vi "Text control 2 v1.9.vi"() -> ()   [LabVIEW 2016]
panel:
  out "Total iterations":i32
  out "Line running":i32
  in  "byte count":u32=64
  in  "Serial Settings:Serial End Mode for Reads":u16(ring)=2 items=["None", "LastBit", "TermChar"]
  in  "Timeout (ms)":u32=10000
  in  "Enable Termination\nChar (T)":bool=TRUE
  in  "Termination char\n(0xA = '\\n' = LF)\n(0xD = '\\r' = CR)":u8=13 format="%.0x"
  in  "flow control":u16(ring) items=["None"=0, "XON/XOFF"=1, "RTS/CTS"=2, "DTR/DSR"=4]
  in  "stop bits":u16(ring)=10 items=["1.0"=10, "1.5"=15, "2.0"=20]
  in  "parity":u16(ring) items=["None", "Odd", "Even", "Mark", "Space"]
  in  "data bits":u16=8 min=5 max=8 step=1
  in  "VISA resource name":refnum<visa-resource-name>="COM6"
  in  "baud rate":u32=9600
  out "Serial output":string
  out "error out":errorcluster
  in  "Units":bool
  out "Elapsed Time":dbl caption="Elapsed Time (s)"
  out "Ion vs time":cluster{"Y data in":dbl[], "X data in":dbl[]}[](graph)
  out "Ig":dbl format="%.2e"
  out "Id":dbl format="%.2e"
  out "Is":dbl format="%.2e"
  out "I vs Vg":cluster{"Y data in":dbl[], "X data in":dbl[]}[](graph)
  in  "Panel Controls 2":T1={"Emergency Stop"=refnum, "TransGraph Max"=1e-05, "Text/Graph (text=false)"=TRUE, "TransGraph Min"=1e-11} {"TransGraph Min" format="%.2e"; "TransGraph Max" format="%.2e"}
  out "Command running:":string="#output s 0 0 0 -0.008 0.008 0.002"
  in  "Standby":T2
  in  "Full Reset":bool
  in  "SMU4":cluster{"on/off":bool, "Voltage":dbl} {"Voltage" min=-100.0 max=100.0 format="%.2f"}
  in  "Source/Drain Range":u8(slide)=6 max=11 scale=0.0..11.0
  in  "Source/Drain\nRange mode":u16(ring) items=["Auto", "Limited", "Fixed"]
  in  "Gate Range":u8(slide)=6 max=11 scale=0.0..11.0
  in  "Gate Range\nmode":u16(ring) items=["Auto", "Limited", "Fixed"]
  in  "Gate":T3={"Gate Start"=0.0, "Gate Stop"=2.0, "Gate Step (linear only)"=1.0, "Gate Compliance"=0.0001, "Gate PComp"=0.0, "Range mode"=0, "Range"=6} {"Range" max=11 scale=0.0..11.0; "Range mode" items=["Auto", "Limited", "Fixed"]; "Gate PComp" format="%^.2e"; "Gate Compliance" format="%^.2e"; "Gate Step (linear only)" format="%^.4e"; "Gate Stop" format="%^.4e"; "Gate Start" format="%^.4e"}
  in  "Drain 2":T4={"Drain Start"=0.0, "Drain Stop"=2.0, "Drain Compliance"=0.0001, "Drain Step"=1.0, "Drain PComp"=0.0, "Range mode"=0, "Range"=6} {"Range" max=11 scale=0.0..11.0; "Range mode" items=["Auto", "Limited", "Fixed"]; "Drain PComp" format="%^.2e"; "Drain Step" format="%^.4e"; "Drain Compliance" format="%^.2e"; "Drain Stop" format="%^.4e"; "Drain Start" format="%^.4e"}
  in  "Timings 2":T5={"integration time"=0, "Short/Long integration time"=0.00064, "hold time (sec)"=0.0, "delay time (sec)"=0.0, "Step Time (0 disables)"=0.0, "sweep method"=0, "Pulse period"=0.005, "Base voltage"=0.0, "Pulse width"=0.0005} {"Pulse width" min=0.0005 max=0.1 step=0.0001 format="%.4f"; "Base voltage" format="%^.4e"; "Pulse period" min=0.005 max=1.0 step=0.0001 format="%.4f"; "sweep method" items=["Continuous", "Pulsed"]; "Step Time (0 disables)" format="%.2f"; "delay time (sec)" format="%.4f"; "hold time (sec)" format="%.4f"; "Short/Long integration time" format="%^.0e"; "integration time" scale=0.0..2.0}
  in  "Panel Controls":T6={"Emergency Stop"=refnum, "TransGraph Max"=1e-05, "Text/Graph (text=false)"=TRUE} {"TransGraph Max" format="%.2e"}
  in  "Interrupt run":bool
  in  "Drain: Compliance":dbl=0.001 format="%.8f"
  in  "Gate: Compliance":dbl=0.001 format="%.8f"
  out "Path":path=path "C:/users/rlp38/09Apr2009LTtesting/test2.txt"
  in  "hold time /s":dbl format="%.2f"
  in  "delay time /s":dbl format="%.2f"
  in  "integration time":u32(slide) max=2 step=1 scale=0.0..2.0
  in  "Integration time (short)":dbl=0.0019 min=8e-05 max=0.0019 step=8e-05 format="%^.0e"
  in  "Integration time (long)":dbl=0.32 min=0.04 max=2.0 step=0.02 format="%.2f"
  in  "Step delay /s":dbl format="%.2f"
  in  "Program":string="#pulsedstressV d 0.03 20 0 0.5 0.0827 5\n#\n#itime s\n#gaterangemode l\n#drainrangemode l\n#pulsed on 0.05 0 0.02\n#transfer d 1 -1 -0.1 -1 -1 0\n#wait-min 1\n#transfer d 1 -1 -0.1 -1 -1 0\n#output d 0 -1 -0.5 0 -1 -0.1\n#transfer d -10 40 1 5 40 35\n#transfer d -10 40 1 5 40 35\n#output d 0 40 20 0 40 1\n#\n#\n#sample 1 0.008 221 6 0.003\n#samplei 400e-6 200 6 0.002 0.1\n#vsu2pulse -10 4\n#\n#stressV 0.016 0.03 2e-4 0.1e-3 11\n#stressI 220e-7 0.08 15\n#transfer s -1 1 0.5 -0.005 0.005 0.005\n#output s 0 0 0 -0.008 0.008 0.002\n"
  # "Syntax:\nitime [s|m|l]\ngaterangemode [a|l|f]\ndrainrangemode [a|l|f]\npulsed [on|off] PulsePeriod(sec) PulseBaseVoltage PulseONWidth(sec)\nstandby [on l off]\nwait NumMilliseconds\nwait-min NumMinutes\n# texthere = comment\ntransfer [s|d] VgStart VgStop VgStep VdStart VdStop VdStep\noutput [s|d] VgStart VgStop VgStep VdStart VdStop VdStep\nsample Vg Vd NumSamples Time(s) SampleInterval(s)\nsamplei Idg NumSamples Time(s) SampleInterval(s) VDGcompliance\n# if in doubt use SampleInterval(s) = 0.004\nstressV VG VD IGcompliance IDcompliance Duration(sec)\nstressI IDG VDGcompliance Duration(sec)\nvsu2pulse Bias Duration(s)\npulsedstressV [s|d] VEstop VgON VgOFF Period(s) PulseONwidth(s) Vd\nsample-fpp Vg Vd NumSamples Time\nresample-fpp Vg Vd\ntransfer-fpp [s|d] VgStart VgStop VgStep VdStart VdStop VdStep\noutput-fpp [s|d] VgStart VgStop VgStep VdStart VdStop VdStep\nserial SerialPortCommand"
  # "Time"
  # "Sec"
  # "Min"
  # "100 samples is approx 13s with medium integration"
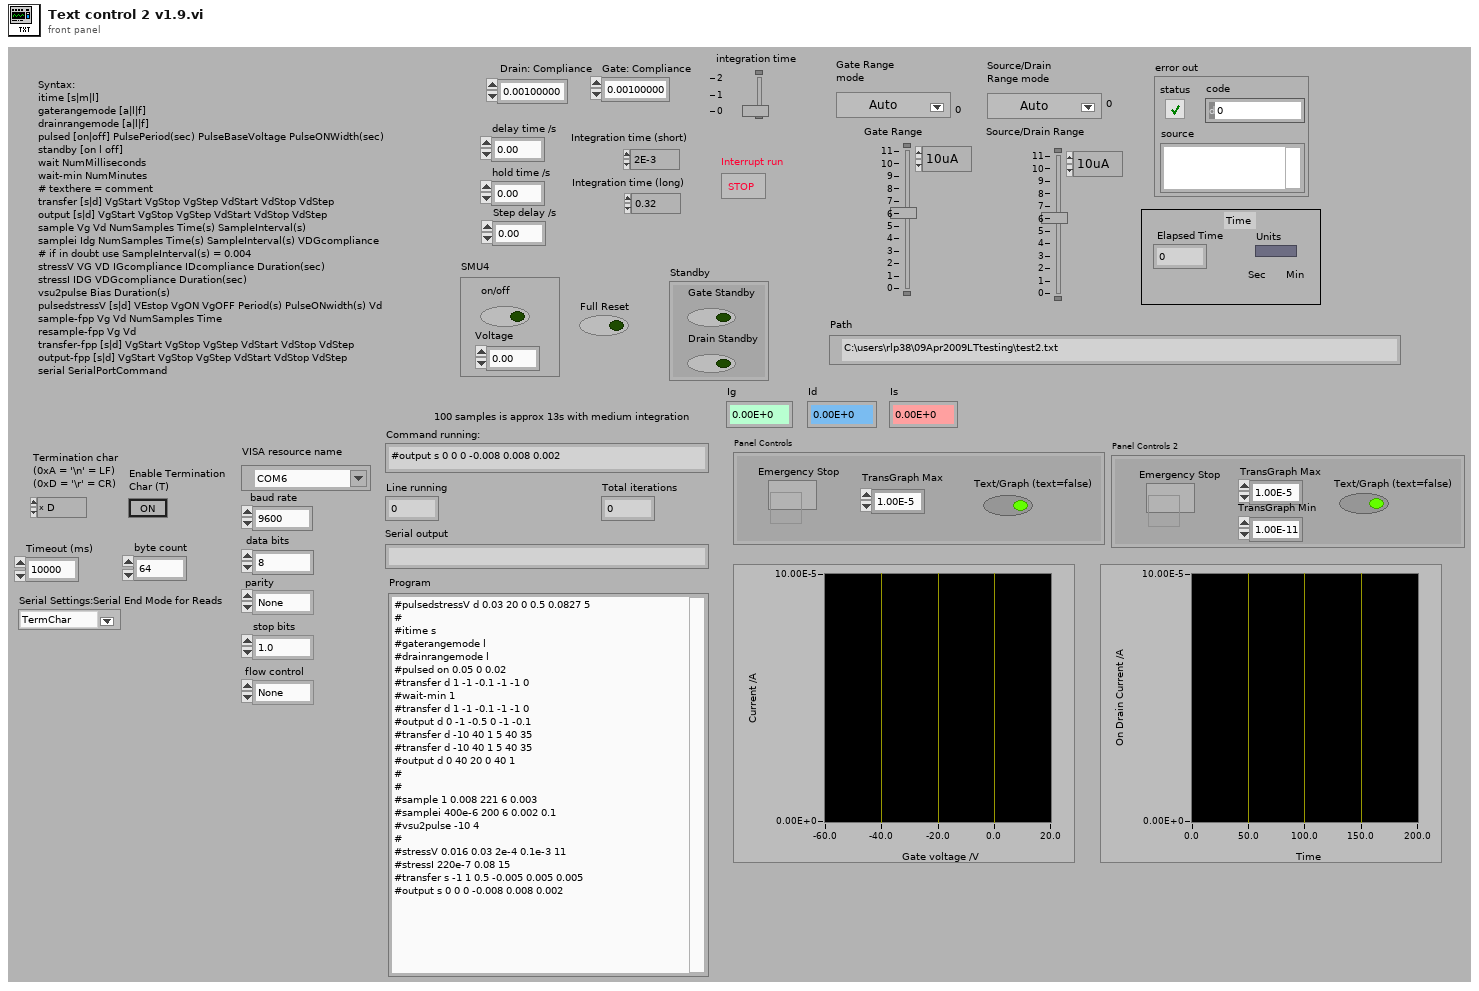
[diagram p1: front panel]
types:
  T1 = cluster{"Emergency Stop":refnum<vi>, "TransGraph Max":dbl, "Text/Graph (text=false)":bool, "TransGraph Min":dbl}
  T2 = cluster{"Gate Standby":bool, "Drain Standby":bool}
  T3 = cluster{"Gate Start":dbl, "Gate Stop":dbl, "Gate Step (linear only)":dbl, "Gate Compliance":dbl, "Gate PComp":dbl, "Range mode":u16, "Range":u8}
  T4 = cluster{"Drain Start":dbl, "Drain Stop":dbl, "Drain Compliance":dbl, "Drain Step":dbl, "Drain PComp":dbl, "Range mode":u16, "Range":u8}
  T5 = cluster{"integration time":u32, "Short/Long integration time":dbl, "hold time (sec)":dbl, "delay time (sec)":dbl, "Step Time (0 disables)":dbl, "sweep method":u16, "Pulse period":dbl, "Base voltage":dbl, "Pulse width":dbl}
  T6 = cluster{"Emergency Stop":refnum<vi>, "TransGraph Max":dbl, "Text/Graph (text=false)":bool}
  T7 = enum16{"open", "replace", "create", "open or create", "replace or create", "replace or create with confirmation"}
  T8 = cluster{"V2 Start":dbl, "V2 Step":dbl, "Number of points":i32}
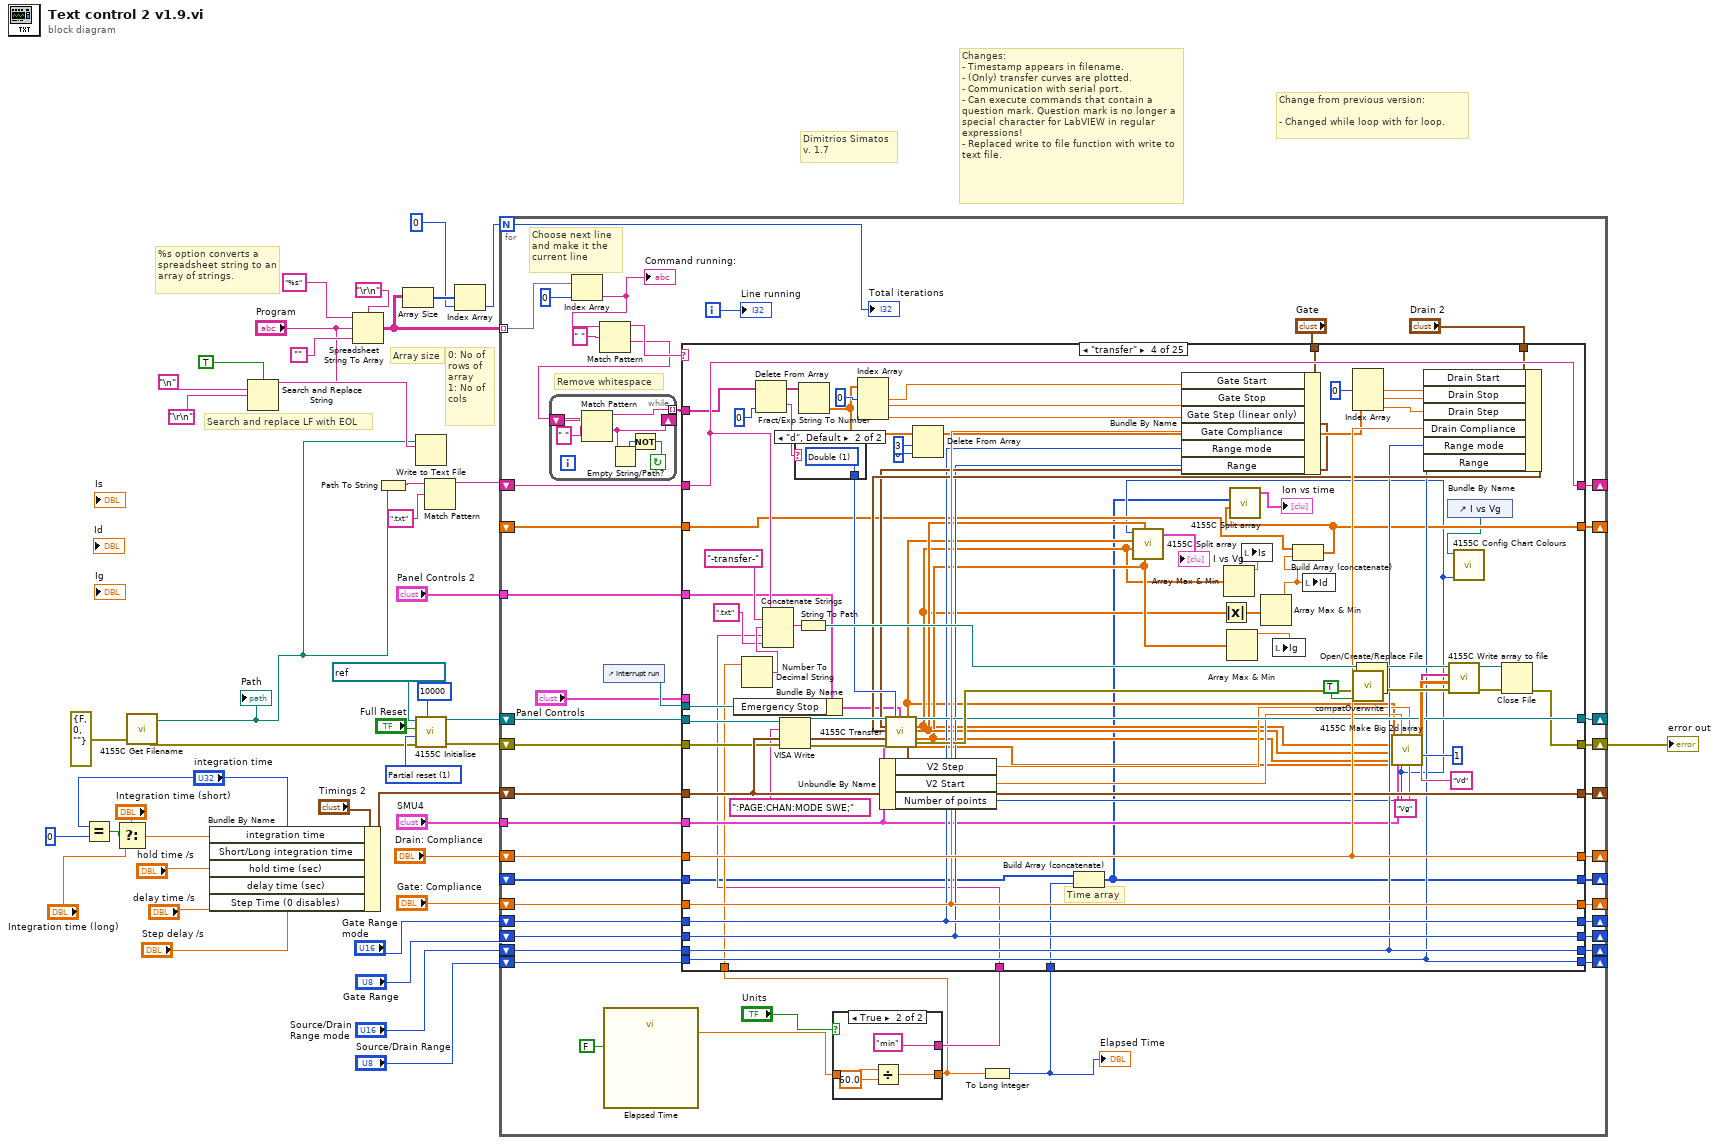
[diagram p0: block diagram]
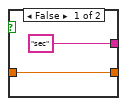
[diagram p2: hidden frame]
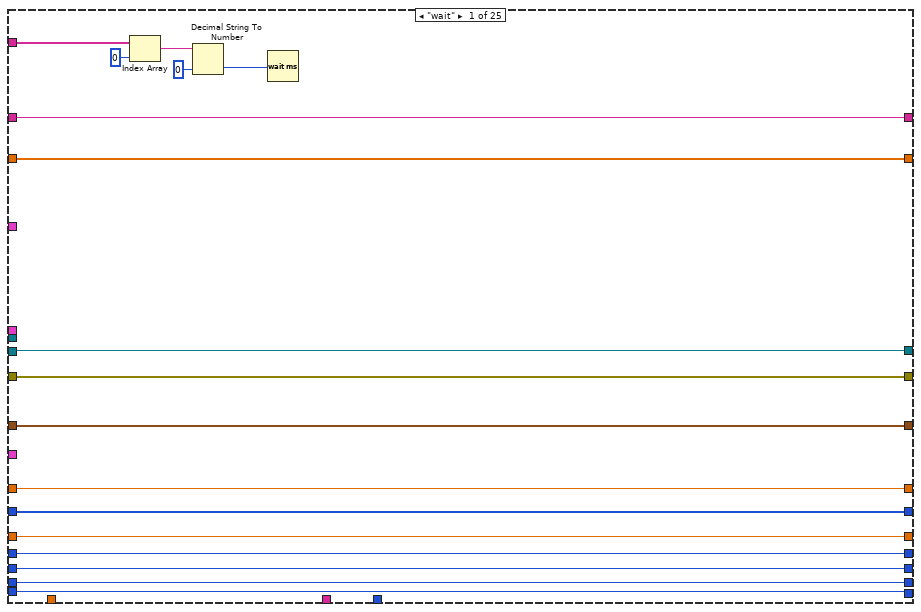
[diagram p3: hidden frame]
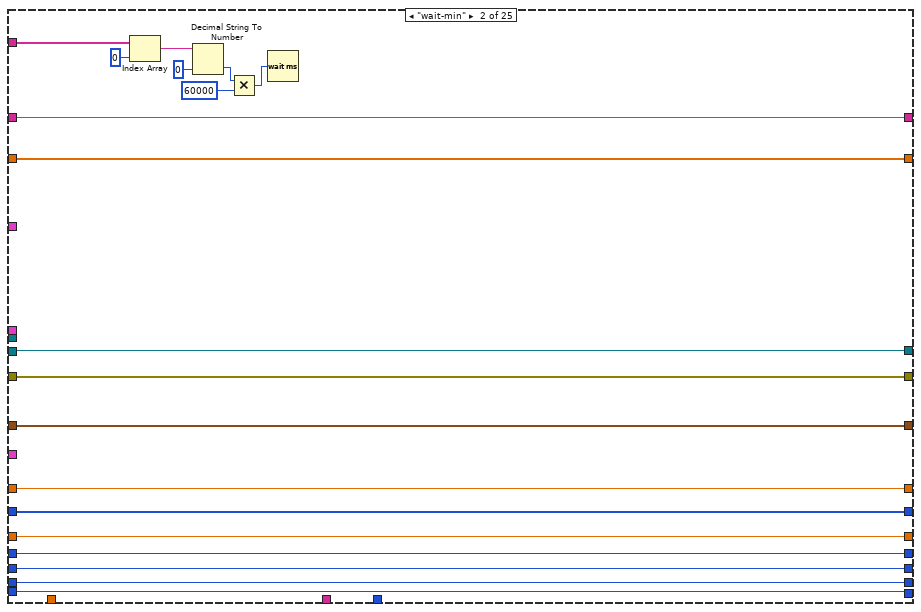
[diagram p4: hidden frame]
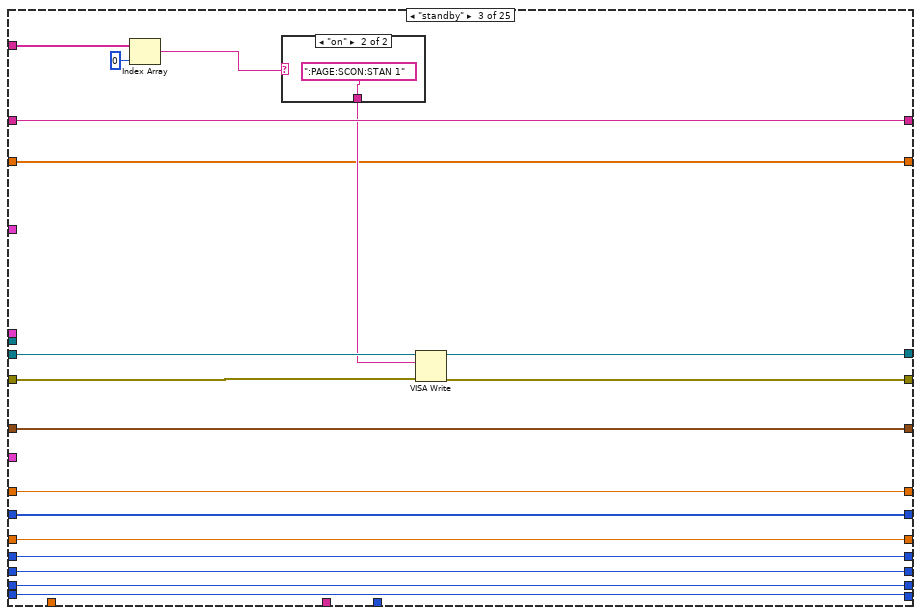
[diagram p5: hidden frame]
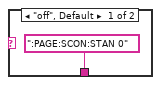
[diagram p6: hidden frame]
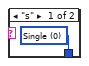
[diagram p7: hidden frame]
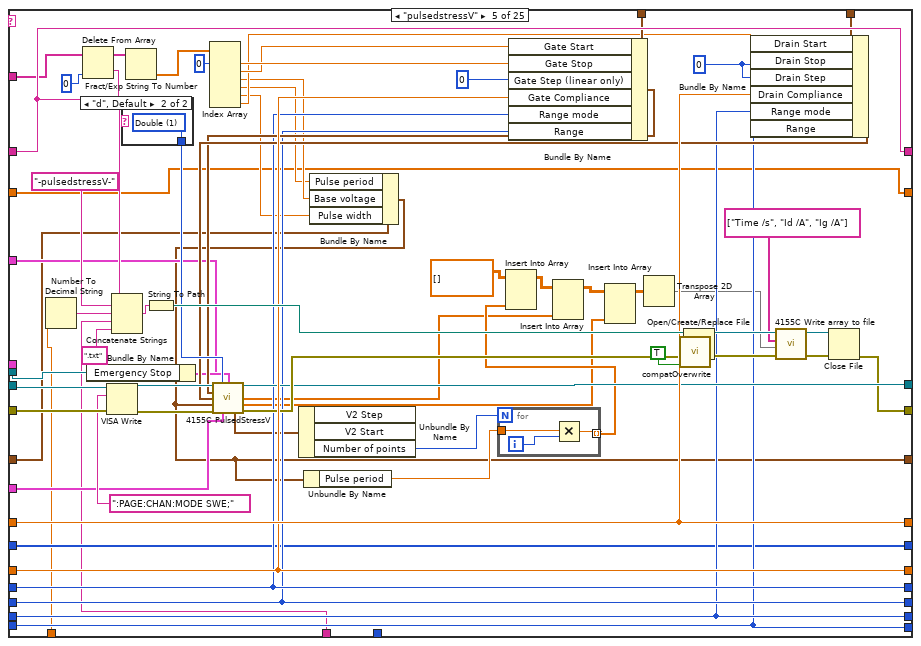
[diagram p8: hidden frame]
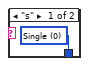
[diagram p9: hidden frame]
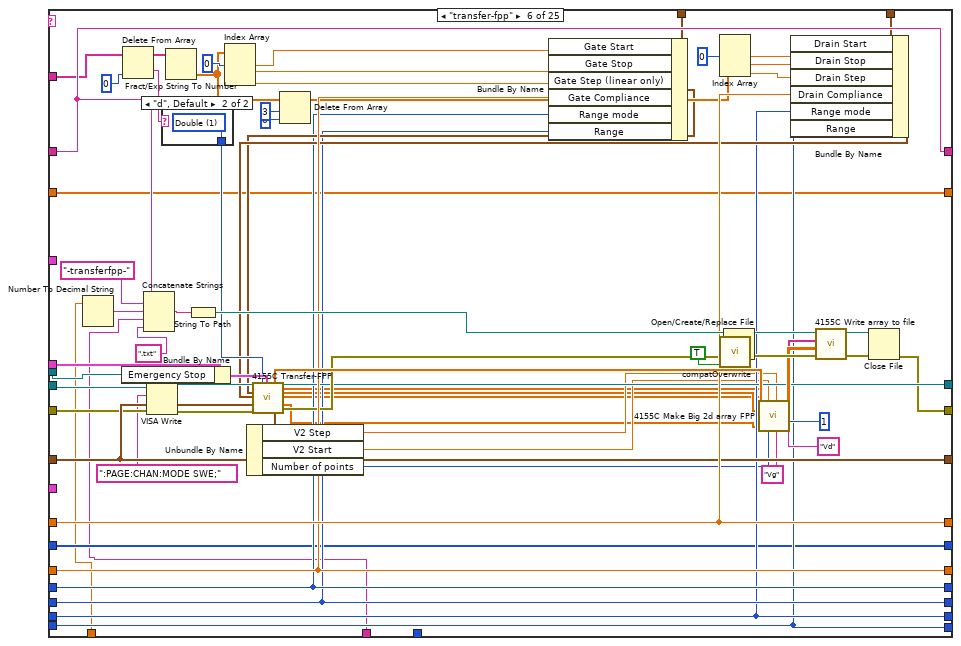
[diagram p10: hidden frame]
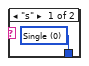
[diagram p11: hidden frame]
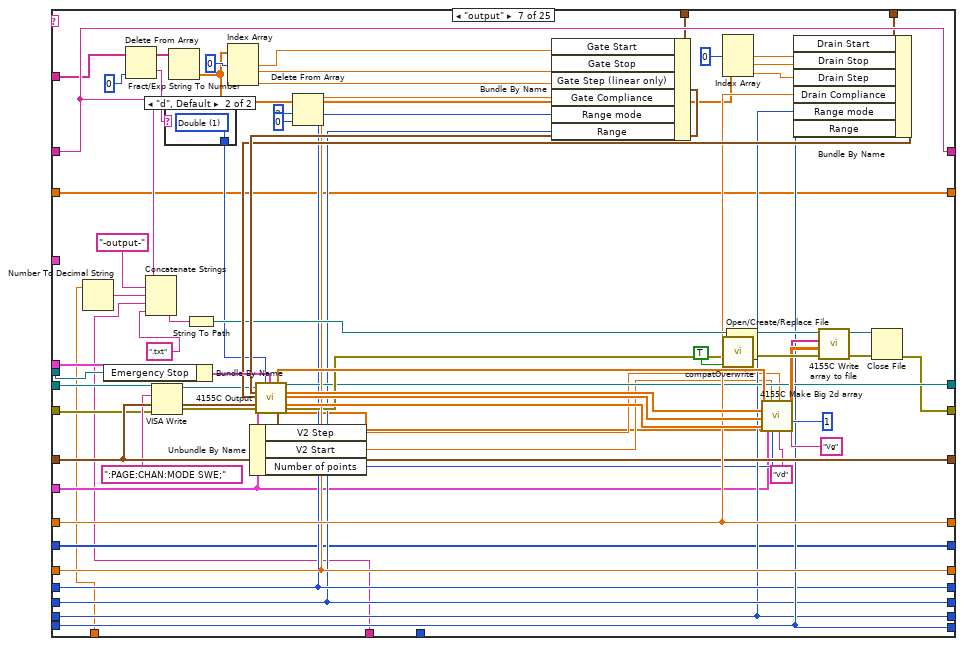
[diagram p12: hidden frame]
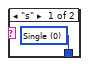
[diagram p13: hidden frame]
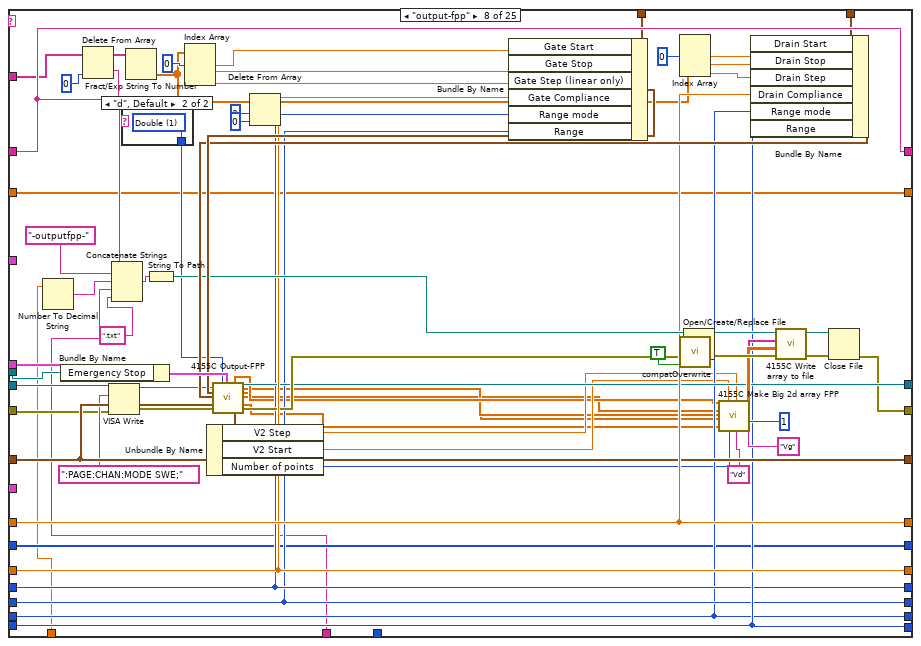
[diagram p14: hidden frame]
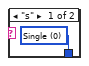
[diagram p15: hidden frame]
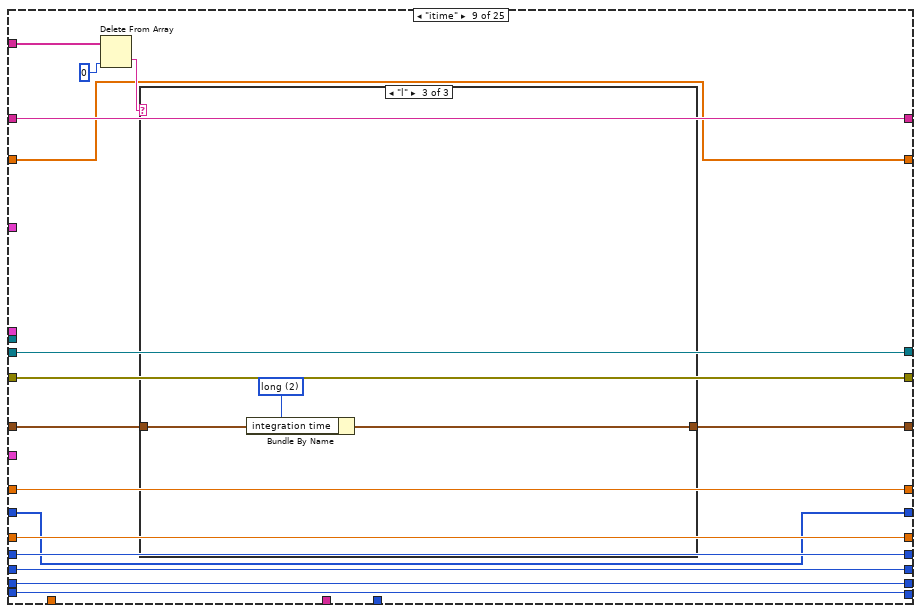
[diagram p16: hidden frame]
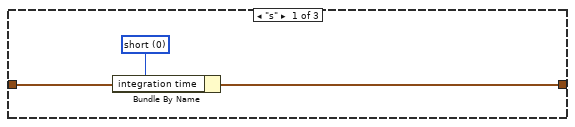
[diagram p17: hidden frame]
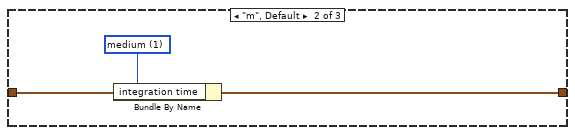
[diagram p18: hidden frame]
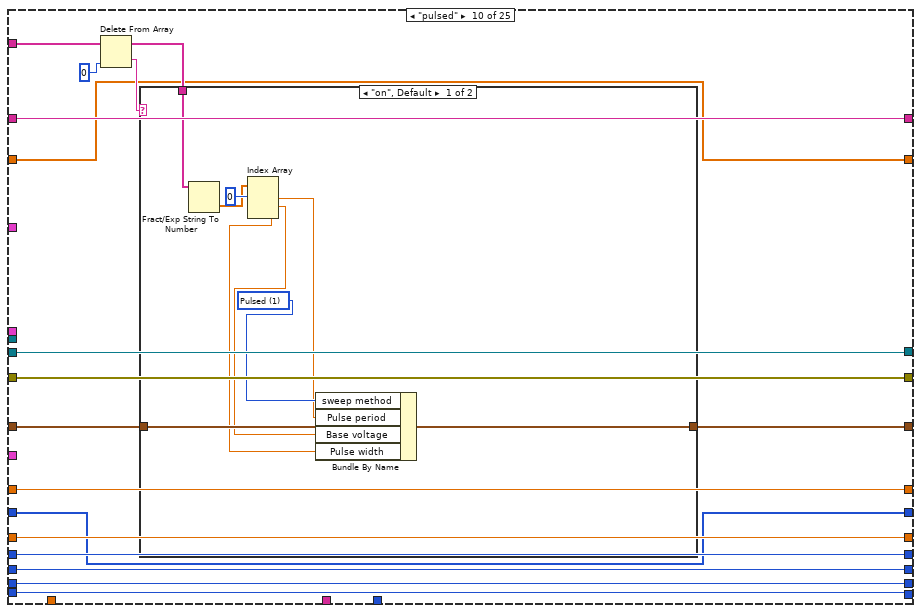
[diagram p19: hidden frame]
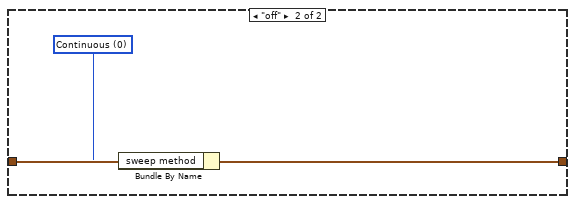
[diagram p20: hidden frame]
diagram:
  w35 = u16 1 items=["Reset All", "Partial reset"] ("Type of reset")
  # "Array size"
  # "%s option converts a spreadsheet string to an array of strings."
  # "0: No of rows of array\n1: No of cols"
  # "Change from previous version:\n\n- Changed while loop with for loop."
  # "Dimitrios Simatos\nv. 1.7"
  # "Changes:\n- Timestamp appears in filename.\n- (Only) transfer curves are plotted.\n- Communication with serial port.\n- Can execute commands that contain a question mark. Question mark is no longer a special character for LabVIEW in regular expressions!\n- Replaced write to file function with write to text file."
  # "Search and replace LF with EOL"
  n1 = Equal?(x="integration time", y=u32 0) -> (x = y?=w39:bool)
  n2 = Select(t="Integration time (short)", s=w39, f="Integration time (long)") -> (s? t:f=w43:dbl)
  n3 = call "4155C Get Filename.vi"("error in (no error)"=errorcluster {"status"=FALSE, "code"=0, "source"=""}) -> ("error out"=w30:errorcluster, "path"=w14:path)  [unwired: 2 in, 1 out]
  "Path" <- w14
  n4 = Bundle By Name(cluster="Timings 2", "integration time"="integration time", "Short/Long integration time"=w43, "hold time (sec)"="hold time /s", "delay time (sec)"="delay time /s", "Step Time (0 disables)"="Step delay /s") -> (w27:T5)
  n5 = Search and Replace String(replace all?=TRUE ("replace all? (F)"), input string="Program", search string="\n", replace string="\r\n") -> (result string=w17:string)  [unwired: 4 in, 3 out]
  n6 = Spreadsheet String To Array(delimiter (Tab)="\r\n", format string="%s", spreadsheet string="Program", array type (2D Dbl)="") -> (array=w2:string[][])
  n7 = Path To String(path=w14) -> (string=w13:string)
  n8 = Array Size(array=w2) -> (size(s)=w7:i32[])
  n9 = Write to Text File(file (use dialog)=w14, text=w17) -> ()  [unwired: 2 in, 3 out]
  n10 = call "4155C Initialise.vi"("VISA resource name in"=refnum<visa-resource-name> "GPIB0::14::INSTR", "Reset"="Full Reset", "Type of reset"=w35, "error in (no error)"=w30, "VISA Timeout Value"=u32 10000) -> ("VISA Resource Name out"=w29:refnum<visa-resource-name>, "error out"=w28:errorcluster)
  n11 = Match Pattern(string=w13, regular expression=".txt") -> (before substring=w12:string)  [unwired: 1 in, 3 out]
  n12 = Index Array(array=w7, index=0) -> (element=w5:i32)
  n13 = for {
    N: w5 -> [w45]
    tunnel: "SMU4" -> [w61]
    shift-left: "Source/Drain Range" -> [w66]
    shift-right: [w62] -> _
    shift-left: "Source/Drain\nRange mode" -> [w67]
    shift-right: [w63] -> _
    shift-left: "Gate Range" -> [w68]
    shift-right: [w64] -> _
    shift-left: "Gate Range\nmode" -> [w69]
    shift-right: [w65] -> _
    shift-left: "Gate: Compliance" -> [w80]
    shift-right: [w75] -> _
    shift-left: "Drain: Compliance" -> [w81]
    shift-right: [w76] -> _
    shift-left: w27 -> [w82]
    shift-right: [w77] -> _
    shift-left: w28 -> [w83]
    shift-right: [w78] -> w9
    shift-left: w29 -> [w84]
    shift-right: [w79] -> _
    shift-left: w12 -> [w85]
    shift-right: [w74] -> _
    tunnel: "Panel Controls 2" -> [w60]
    shift-right: [w59] -> _
    shift-left: _ -> [w58]
    shift-right: [w53] -> _
    shift-left: _ -> [w52]
    tunnel: w2 -> [w48] mode=indexing
    i -> [w46]
    # "Choose next line\nand make it the current line"
    # "Remove whitespace"
    n14 = Index Array(array=w48, index=0 ("line index")) -> (element=w49:string)
    "Command running:" <- w49
    n15 = Match Pattern(string=w49, regular expression=" ") -> (before substring=w88:string, after substring=w87:string)  [unwired: 1 in, 2 out]
    n16 = while {
      tunnel: [w96] -> w86 mode=indexing
      shift-left: w87 -> [w98]
      shift-right: [w97] -> _
      stop <- w100 continue-if-true
      n17 = Match Pattern(string=w98, regular expression=" ") -> (before substring=w96:string, after substring=w97:string)  [unwired: 1 in, 2 out]
      n18 = Empty String/Path?(string/path=w97) -> (empty?=w101:bool)
      n19 = Not(x=w101) -> (.not. x?=w100:bool)
    }
    n20 = control-ref of="Interrupt run"() -> (w73:refnum<vi>)
    n21 = call "Elapsed Time"("Auto Reset"=FALSE) -> ("Elapsed Time (s)"=w54:dbl)  [unwired: 11 in, 7 out]
    n22 = case shown="True" "Units" {
      tunnel: ["sec" "min"] -> w55
      tunnel: [w90 w94] -> w51
      tunnel: w54 -> [w90 w93]
      frame False {
      }
      frame True {
        n23 = Divide(x=w93, y=60.0) -> (x/y=w94:dbl)
      }
    }
    n24 = To Long Integer(number=w51) -> (32bit integer=w50:i32)
    "Elapsed Time" <- w50
    n25 = case shown="\"transfer\"" w88 {
      tunnel: w86 -> [w118 w137 w155 w219 w290 w359 w426 w501 w539 w565 w592 w617 w638 w652 _ _ w756 w817 _ w882 w926 w968 w1038 w1100 w1107]
      tunnel: w85 -> [w113 w133 w153 w227 w297 w367 w434 w509 w528 w554 w584 w610 w632 w645 w664 w706 w734 w799 w830 w869 w913 w956 w1032 w1096 w1109]
      tunnel: w84 -> [w112 w132 w144 w197 w281 w336 w402 w477 w529 w555 w585 w611 w633 w646 w669 w708 w762 w823 w834 w888 w932 w974 w1044 w1054 w1113]
      tunnel: w83 -> [w111 w131 w143 w196 w280 w335 w399 w474 w530 w556 w586 w612 w634 w647 w668 w679 w761 w822 w833 w887 w931 w973 w1043 w1053 w1112]
      tunnel: w82 -> [w110 w130 w152 w223 w256 w363 w430 w505 w538 w564 w583 w609 w631 w644 w667 w703 w725 w791 w839 w862 w906 w949 w1031 w1095 w1114]
      tunnel: w81 -> [w109 w129 w151 w225 w295 w365 w432 w507 w537 w563 w591 w616 w637 w651 w666 w688 w760 w821 w842 w886 w930 w972 w1042 w1104 w1115]
      tunnel: w80 -> [w108 w128 w150 w224 w294 w364 w431 w506 w536 w562 w590 w615 w636 w650 w665 w689 w735 w800 w841 w870 w914 w957 w1033 w1097 w1117]
      tunnel: [w112 w132 w142 w221 w292 w361 w428 w503 w529 w555 w585 w611 w633 w646 w669 w708 w726 w773 w832 w863 w907 w950 w984 w1056 w1113] -> w79
      tunnel: [w111 w131 w141 w220 w291 w360 w427 w502 w530 w556 w586 w612 w634 w647 w668 w678 w736 w774 w831 w871 w915 w958 w983 w1055 w1111] -> w78
      tunnel: [w110 w130 w152 w223 w252 w363 w430 w505 w531 w557 w583 w609 w631 w644 w667 w703 w725 w791 w839 w862 w906 w949 w1031 w1095 w1114] -> w77
      tunnel: [w109 w129 w151 w225 w295 w365 w432 w507 w537 w563 w591 w616 w637 w651 w666 w688 w760 w821 w842 w886 w930 w972 w1042 w1104 w1115] -> w76
      tunnel: [w108 w128 w150 w224 w294 w364 w431 w506 w536 w562 w590 w615 w636 w650 w665 w689 w735 w800 w841 w870 w914 w957 w1033 w1097 w1117] -> w75
      tunnel: [w113 w133 w153 w227 w297 w367 w434 w509 w528 w554 w584 w610 w632 w645 w664 w706 w734 w799 w830 w869 w913 w956 w1032 w1096 w1109] -> w74
      tunnel: w73 -> [_ _ _ w230 w301 w372 w442 w513 _ _ _ _ _ _ _ _ w731 w796 _ w868 w912 w955 w1004 w1072 _]
      tunnel: "Gate" -> [_ _ _ w206 w284 w346 w413 w488 _ _ _ _ _ _ _ _ _ _ _ _ _ _ _ _ _]
      tunnel: "Drain 2" -> [_ _ _ w205 w283 w345 w412 w487 _ _ _ _ _ _ _ _ _ _ _ _ _ _ _ _ _]
      tunnel: "Panel Controls" -> [_ _ _ _ _ w344 w411 w486 _ _ _ _ _ _ _ _ _ _ _ _ _ _ _ _ _]
      tunnel: w69 -> [w107 w127 w149 w190 w274 w329 w397 w472 w535 w561 _ w608 w630 w643 w663 w690 w721 w787 w835 w858 w902 w945 w1027 w1091 w1118]
      tunnel: w68 -> [w106 w126 w148 w189 w273 w328 w396 w471 w534 w560 w589 _ w621 w649 w662 w691 w722 w788 w836 w859 w903 w946 w1028 w1092 w1119]
      tunnel: w67 -> [w105 w125 w147 w188 w272 w327 w395 w470 w533 w559 w588 w614 w635 _ w661 w692 w723 w789 w837 w860 w904 w947 w1029 w1093 w1120]
      tunnel: w66 -> [w104 w124 w146 w187 w271 w326 w398 w473 w532 w558 w587 w613 _ w648 w660 w693 w724 w790 w838 w861 w905 w948 w1030 w1094 w1121]
      tunnel: [w107 w127 w149 w190 w274 w329 w397 w472 w535 w561 w582 w608 w630 w643 w663 w690 w721 w787 w835 w858 w902 w945 w1027 w1091 w1118] -> w65
      tunnel: [w106 w126 w148 w189 w273 w328 w396 w471 w534 w560 w589 w600 w621 w649 w662 w691 w722 w788 w836 w859 w903 w946 w1028 w1092 w1119] -> w64
      tunnel: [w105 w125 w147 w188 w272 w327 w395 w470 w533 w559 w588 w614 w635 w642 w661 w692 w723 w789 w837 w860 w904 w947 w1029 w1093 w1120] -> w63
      tunnel: [w104 w124 w146 w187 w271 w326 w398 w473 w532 w558 w587 w613 w622 w648 w660 w693 w724 w790 w838 w861 w905 w948 w1030 w1094 w1121] -> w62
      tunnel: w61 -> [_ _ _ w182 w268 _ w390 _ _ _ _ _ _ _ _ _ _ _ _ _ _ _ _ _ _]
      tunnel: w60 -> [_ _ _ w180 w267 _ _ _ _ _ _ _ _ _ _ _ _ _ _ _ _ _ _ _ _]
      tunnel: [w103 w120 w139 w169 w244 w316 w387 w459 w527 w552 w581 w599 w620 w641 w659 w674 w713 w771 w829 w847 w895 w939 w981 w1049 w1110] -> w59
      tunnel: w58 -> [w103 w120 w139 w168 w244 w316 w387 w459 w527 w552 w581 w599 w620 w641 w659 w674 w713 w771 w829 w847 w895 w939 w981 w1049 w1110]
      tunnel: w51 -> [_ _ _ w164 w241 w314 w384 w456 _ _ _ _ _ _ _ w672 w711 w768 _ w844 w892 w936 w978 w1045 _]
      tunnel: w55 -> [_ _ _ w161 w240 w312 w383 w455 _ _ _ _ _ _ _ w670 w709 w767 _ w843 w891 w935 w977 w1046 _]
      tunnel: w50 -> [_ _ _ w158 _ _ _ _ _ _ _ _ _ _ _ _ _ _ _ _ _ _ _ _ _]
      tunnel: [w102 w119 w138 w160 w243 w315 w386 w458 w526 w551 w580 w598 w619 w640 w658 w673 w712 w770 w828 w846 w894 w938 w980 w1048 w1116] -> w53
      tunnel: w52 -> [w102 w119 w138 w159 w243 w315 w386 w458 w526 w551 w580 w598 w619 w640 w658 w673 w712 w770 w828 w846 w894 w938 w980 w1048 w1116]
      frame "wait" {
        n26 = Index Array(array=w118, index=0 ("Index")) -> (element=w116:string)
        n27 = Decimal String To Number(string=w116, default (0L)=u32 0) -> (number=w115:u32)  [unwired: 1 in, 1 out]
        n28 = Wait (ms)(milliseconds to wait=w115) -> ()  [unwired: 1 out]
      }
      frame "wait-min" {
        n29 = Index Array(array=w137, index=0 ("Index")) -> (element=w135:string)
        n30 = Decimal String To Number(string=w135, default (0L)=u32 0) -> (number=w123:u32)  [unwired: 1 in, 1 out]
        n31 = Multiply(x=w123, y=u32 60000) -> (x*y=w122:u32)
        n32 = Wait (ms)(milliseconds to wait=w122) -> ()  [unwired: 1 out]
      }
      frame "standby" {
        n33 = Index Array(array=w155, index=0 ("Index")) -> (element=w145:string)
        n34 = case shown="\"on\"" w145 {
          tunnel: [":PAGE:SCON:STAN 0" ":PAGE:SCON:STAN 1"] -> w140
          frame "off", Default {
          }
          frame "on" {
          }
        }
        n35 = VISA Write(VISA resource name=w144, write buffer=w140, error in (no error)=w143) -> (VISA resource name out=w142:refnum<visa-resource-name>, error out=w141:errorcluster)  [unwired: 1 out]
      }
      frame "transfer" {
        # "Time array"
        n36 = Bundle By Name(cluster=w180, "Emergency Stop"=w230) -> (w181:T1)
        n37 = Number To Decimal String(number=w164) -> (decimal integer string=w163:string)  [unwired: 1 in]
        n38 = Delete From Array(array=w219, index=0 ("Index")) -> (deleted portion=w217:string, array with subset deleted=w216:string[])  [unwired: 1 in]
        n39 = Concatenate Strings(w227, "-transfer-" ("Prefix"), w163, w161, ".txt" ("Suffix")) -> (w229:string)
        n40 = VISA Write(VISA resource name=w197, write buffer=":PAGE:CHAN:MODE SWE;" ("write buffer (\"\")"), error in (no error)=w196) -> (VISA resource name out=w194:refnum<visa-resource-name>, error out=w195:errorcluster)  [unwired: 1 out]
        n41 = case shown="\"d\", Default" w217 {
          tunnel: [w238 w239] -> w215
          frame "s" {
            w238 = u16 0 items=["Single", "Double"] ("sweep mode")
          }
          frame "d", Default {
            w239 = u16 1 items=["Single", "Double"] ("sweep mode")
          }
        }
        n42 = String To Path(string=w229) -> (path=w226:path)
        n43 = Fract/Exp String To Number(string=w216) -> (number=w201:dbl[])  [unwired: 3 in, 1 out]
        n44 = Index Array(array=w201, index #1=0 ("Index")) -> (element #1=w214:dbl, element #2=w213:dbl, element #3=w212:dbl)  [unwired: 2 in]
        n45 = Delete From Array(array=w201, length=3 ("Length"), index=0 ("Index")) -> (array with subset deleted=w199:dbl[])  [unwired: 1 out]
        n46 = Build Array (concatenate)(w159, w158) -> (w160:i32[])
        n47 = Bundle By Name(cluster=w206, "Gate Start"=w214, "Gate Stop"=w213, "Gate Step (linear only)"=w212, "Gate Compliance"=w224, "Range mode"=w190, "Range"=w189) -> (w191:T3)
        n48 = Index Array(array=w199, index #1=0 ("Index")) -> (element #1=w209:dbl, element #2=w208:dbl, element #3=w207:dbl)  [unwired: 2 in]
        n49 = call <vilib>:"compatOverwrite.vi"("overwrite (F)"=TRUE) -> ("overwrite?"=w179:T7)
        n50 = Bundle By Name(cluster=w205, "Drain Start"=w209, "Drain Stop"=w208, "Drain Step"=w207, "Drain Compliance"=w225, "Range mode"=w188, "Range"=w187) -> (w192:T4)
        n51 = call "4155C Transfer.vi"("VISA resource name in"=w194, "Gate"=w191, "Drain"=w192, "Timings"=w223, "error in (no error)"=w195, "SMU4"=w182, "sweep mode"=w215, "Panel Controls"=w181) -> ("VG"=w170:dbl[], "Outparams"=w186:T8, "VISA Resource Name out"=w221:refnum<visa-resource-name>, "IS"=w172:dbl[], "ID"=w177:dbl[], "IG"=w173:dbl[], "error out"=w222:errorcluster, "SMU4"=w183:dbl[])  [unwired: 12 in]
        n52 = Unbundle By Name(w186) -> ("V2 Step"=w185:dbl, "V2 Start"=w184:dbl, "Number of points"=w166:i32)
        n53 = call "4155C Split array.vi"("Number of VAR2 steps"=w166, "Y2 data in"=w177, "X data in"=w170, "Y1 data in"=w172, "Y3 data in"=w173) -> ("Array of clusters"=→"I vs Vg":cluster{"Y data in":dbl[], "X data in":dbl[]}[])  [unwired: 2 in, 1 out]
        n54 = Absolute Value(x=w172) -> (abs(x)=w176:dbl[])
        n55 = Array Max & Min(array=w172) -> (max value=w174:dbl)  [unwired: 3 out]
        n56 = Array Max & Min(array=w173) -> (max value=w175:dbl)  [unwired: 3 out]
        n57 = local write "Is"(w174) -> ()
        n58 = Array Max & Min(array=w176) -> (max value=w167:dbl)  [unwired: 3 out]
        n59 = local write "Ig"(w175) -> ()
        n60 = Build Array (concatenate)(w168, w167) -> (w169:dbl[])
        n61 = call "4155C Split array.vi"("X data in"=w160, "Y1 data in"=w169) -> ("Array of clusters"=→"Ion vs time":cluster{"Y data in":dbl[], "X data in":dbl[]}[])  [unwired: 5 in, 1 out]
        n62 = local write "Id"(w167) -> ()
        n63 = Open/Create/Replace File(file path (use dialog)=w226, error in=w222, operation (0:open)=w179) -> (refnum out=w235:refnum<file>, error out=w236:errorcluster)  [unwired: 3 in, 1 out]
        n64 = call "4155C Make Big 2d array.vi"("1D Var1"=w170, "1d IS"=w172, "1d ID"=w177, "1d IG"=w173, "1d SMU4"=w183, "SMU4"=w182, "VAR2 START"=w184, "Number of VAR2 steps"=w166, "VAR2 STEP"=w185, "VAR1 Name"="Vg", "Decimal places in header"=i8 1, "VAR2 Name"="Vd") -> ("Header array"=w231:string[], "Data array"=w232:dbl[][])  [unwired: 14 in]
        n65 = control-ref of="I vs Vg"() -> (w165:refnum<vi>)
        n66 = call "4155C Write array to file.vi"("Byte Stream File Refnum"=w235, "Header"=w231, "Data Array"=w232, "error in (no error)"=w236) -> ("dup refnum"=w233:refnum<file>, "error out"=w234:errorcluster)  [unwired: 1 in]
        n67 = call "4155C Config Chart Colours.vi"("Numeric"=w166, "XY Graph 2"=w165) -> ()  [unwired: 6 in]
        n68 = Close File(refnum=w233, error in=w234) -> (error out=w220:errorcluster)  [unwired: 1 out]
      }
      frame "pulsedstressV" {
        w250 = 0
        n69 = Number To Decimal String(number=w241) -> (decimal integer string=w298:string)  [unwired: 1 in]
        n70 = Delete From Array(array=w290, index=0 ("Index")) -> (deleted portion=w288:string, array with subset deleted=w287:string[])  [unwired: 1 in]
        n71 = Bundle By Name(cluster=w267, "Emergency Stop"=w301) -> (w269:T1)
        n72 = VISA Write(VISA resource name=w281, write buffer=":PAGE:CHAN:MODE SWE;" ("write buffer (\"\")"), error in (no error)=w280) -> (VISA resource name out=w278:refnum<visa-resource-name>, error out=w279:errorcluster)  [unwired: 1 out]
        n73 = Concatenate Strings(w297, "-pulsedstressV-" ("Substring"), w298, w240, ".txt" ("Substring")) -> (w300:string)
        n74 = case shown="\"d\", Default" w288 {
          tunnel: [w310 w311] -> w286
          frame "s" {
            w310 = u16 0 items=["Single", "Double"] ("sweep mode")
          }
          frame "d", Default {
            w311 = u16 1 items=["Single", "Double"] ("sweep mode")
          }
        }
        n75 = Fract/Exp String To Number(string=w287) -> (number=w282:dbl[])  [unwired: 3 in, 1 out]
        n76 = String To Path(string=w300) -> (path=w296:path)
        n77 = Index Array(array=w282, index #1=0 ("Index")) -> (element #1=w259:dbl, element #2=w258:dbl, element #3=w255:dbl, element #4=w254:dbl, element #5=w253:dbl, element #6=w257:dbl)  [unwired: 5 in]
        n78 = Bundle By Name(cluster=w256, "Pulse period"=w254, "Base voltage"=w255, "Pulse width"=w253) -> (w252:T5)
        n79 = Unbundle By Name(w252) -> ("Pulse period"=w260:dbl)
        n80 = Bundle By Name(cluster=w284, "Gate Start"=w258, "Gate Stop"=w259, "Gate Step (linear only)"=0, "Gate Compliance"=w294, "Range mode"=w274, "Range"=w273) -> (w275:T3)
        n81 = call <vilib>:"compatOverwrite.vi"("overwrite (F)"=TRUE) -> ("overwrite?"=w245:T7)
        n82 = Bundle By Name(cluster=w283, "Drain Start"=w257, "Drain Stop"=w250, "Drain Step"=w250, "Drain Compliance"=w295, "Range mode"=w272, "Range"=w271) -> (w276:T4)
        n83 = call "4155C PulsedStressV.vi"("VISA resource name in"=w278, "sweep mode"=w286, "Panel Controls"=w269, "Gate"=w275, "Drain"=w276, "Timings"=w252, "error in (no error)"=w279, "SMU4"=w268) -> ("VISA Resource Name out"=w292:refnum<visa-resource-name>, "ID"=w248:dbl[], "IG"=w246:dbl[], "Outparams"=w270:T8, "error out"=w293:errorcluster)  [unwired: 3 in]
        n84 = Unbundle By Name(w270) -> ("Number of points"=w247:i32)  [unwired: 2 out]
        n85 = for {
          N: w247 -> [_]
          tunnel: [w307] -> w249 mode=indexing
          tunnel: w260 -> [w309]
          i -> [w308]
          n86 = Multiply(x=w309, y=w308) -> (x*y=w307:dbl)
        }
        n87 = Insert Into Array(array=dbl[][] [] ("Input Array"), new element=w249) -> (w261:dbl[][])  [unwired: 2 in]
        n88 = Insert Into Array(array=w261, new element=w248) -> (w266:dbl[][])  [unwired: 2 in]
        n89 = Insert Into Array(array=w266, new element=w246) -> (w265:dbl[][])  [unwired: 2 in]
        n90 = Transpose 2D Array(2D array=w265) -> (transposed array=w264:dbl[][])
        n91 = Open/Create/Replace File(file path (use dialog)=w296, error in=w293, operation (0:open)=w245) -> (refnum out=w304:refnum<file>, error out=w305:errorcluster)  [unwired: 3 in, 1 out]
        n92 = call "4155C Write array to file.vi"("Byte Stream File Refnum"=w304, "Header"=string[] ["Time /s", "Id /A", "Ig /A"], "Data Array"=w264, "error in (no error)"=w305) -> ("dup refnum"=w302:refnum<file>, "error out"=w303:errorcluster)  [unwired: 1 in]
        n93 = Close File(refnum=w302, error in=w303) -> (error out=w291:errorcluster)  [unwired: 1 out]
      }
      frame "transfer-fpp" {
        n94 = Number To Decimal String(number=w314) -> (decimal integer string=w368:string)  [unwired: 1 in]
        n95 = Bundle By Name(cluster=w344, "Emergency Stop"=w372) -> (w380:T6)
        n96 = Delete From Array(array=w359, index=0 ("Index")) -> (deleted portion=w357:string, array with subset deleted=w356:string[])  [unwired: 1 in]
        n97 = Concatenate Strings(w367, "-transferfpp-" ("Substring"), w368, w312, ".txt" ("Substring")) -> (w370:string)
        n98 = VISA Write(VISA resource name=w336, write buffer=":PAGE:CHAN:MODE SWE;" ("write buffer (\"\")"), error in (no error)=w335) -> (VISA resource name out=w333:refnum<visa-resource-name>, error out=w334:errorcluster)  [unwired: 1 out]
        n99 = case shown="\"d\", Default" w357 {
          tunnel: [w381 w382] -> w355
          frame "s" {
            w381 = u16 0 items=["Single", "Double"] ("sweep mode")
          }
          frame "d", Default {
            w382 = u16 1 items=["Single", "Double"] ("sweep mode")
          }
        }
        n100 = Fract/Exp String To Number(string=w356) -> (number=w340:dbl[])  [unwired: 3 in, 1 out]
        n101 = String To Path(string=w370) -> (path=w366:path)
        n102 = Index Array(array=w340, index #1=0 ("Index")) -> (element #1=w354:dbl, element #2=w353:dbl, element #3=w352:dbl)  [unwired: 2 in]
        n103 = Delete From Array(array=w340, length=3 ("Length"), index=0 ("Index")) -> (array with subset deleted=w338:dbl[])  [unwired: 1 out]
        n104 = Bundle By Name(cluster=w346, "Gate Start"=w354, "Gate Stop"=w353, "Gate Step (linear only)"=w352, "Gate Compliance"=w364, "Range mode"=w329, "Range"=w328) -> (w330:T3)
        n105 = Index Array(array=w338, index #1=0 ("Index")) -> (element #1=w349:dbl, element #2=w348:dbl, element #3=w347:dbl)  [unwired: 2 in]
        n106 = call <vilib>:"compatOverwrite.vi"("overwrite (F)"=TRUE) -> ("overwrite?"=w317:T7)
        n107 = Bundle By Name(cluster=w345, "Drain Start"=w349, "Drain Stop"=w348, "Drain Step"=w347, "Drain Compliance"=w365, "Range mode"=w327, "Range"=w326) -> (w331:T4)
        n108 = call "4155C Transfer-FPP.vi"("VISA resource name in"=w333, "Gate"=w330, "Drain"=w331, "Timings"=w363, "error in (no error)"=w334, "sweep mode"=w355, "Panel Controls"=w380) -> ("VG"=w371:dbl[], "Outparams"=w325:T8, "VISA Resource Name out"=w361:refnum<visa-resource-name>, "Vprobe2"=w321:dbl[], "ID"=w320:dbl[], "IG"=w319:dbl[], "Vprobe1"=w318:dbl[], "error out"=w362:errorcluster)  [unwired: 13 in]
        n109 = Unbundle By Name(w325) -> ("V2 Step"=w324:dbl, "V2 Start"=w323:dbl, "Number of points"=w322:i32)
        n110 = Open/Create/Replace File(file path (use dialog)=w366, error in=w362, operation (0:open)=w317) -> (refnum out=w377:refnum<file>, error out=w378:errorcluster)  [unwired: 3 in, 1 out]
        n111 = call "4155C Make Big 2d array FPP.vi"("1D Var1"=w371, "1d ID"=w320, "1d Vp2"=w321, "1d IG"=w319, "1d Vp1"=w318, "VAR2 START"=w323, "Number of VAR2 steps"=w322, "VAR2 STEP"=w324, "VAR1 Name"="Vg", "Decimal places in header"=i8 1, "VAR2 Name"="Vd") -> ("Header array"=w373:string[], "Data array"=w374:dbl[][])  [unwired: 15 in]
        n112 = call "4155C Write array to file.vi"("Byte Stream File Refnum"=w377, "Header"=w373, "Data Array"=w374, "error in (no error)"=w378) -> ("dup refnum"=w375:refnum<file>, "error out"=w376:errorcluster)  [unwired: 1 in]
        n113 = Close File(refnum=w375, error in=w376) -> (error out=w360:errorcluster)  [unwired: 1 out]
      }
      frame "output" {
        n114 = Number To Decimal String(number=w384) -> (decimal integer string=w435:string)  [unwired: 1 in]
        n115 = Bundle By Name(cluster=w411, "Emergency Stop"=w442) -> (w452:T6)
        n116 = Delete From Array(array=w426, index=0 ("Index")) -> (deleted portion=w424:string, array with subset deleted=w423:string[])  [unwired: 1 in]
        n117 = Concatenate Strings(w434, "-output-" ("Substring"), w435, w383, ".txt" ("Substring")) -> (w437:string)
        n118 = VISA Write(VISA resource name=w402, write buffer=":PAGE:CHAN:MODE SWE;" ("write buffer (\"\")"), error in (no error)=w399) -> (VISA resource name out=w401:refnum<visa-resource-name>, error out=w400:errorcluster)  [unwired: 1 out]
        n119 = case shown="\"d\", Default" w424 {
          tunnel: [w453 w454] -> w422
          frame "s" {
            w453 = u16 0 items=["Single", "Double"] ("sweep mode")
          }
          frame "d", Default {
            w454 = u16 1 items=["Single", "Double"] ("sweep mode")
          }
        }
        n120 = Fract/Exp String To Number(string=w423) -> (number=w405:dbl[])  [unwired: 3 in, 1 out]
        n121 = String To Path(string=w437) -> (path=w433:path)
        n122 = Index Array(array=w405, index #1=0 ("Index")) -> (element #1=w421:dbl, element #2=w420:dbl, element #3=w419:dbl)  [unwired: 2 in]
        n123 = Delete From Array(array=w405, length=3 ("Length"), index=0 ("Index")) -> (array with subset deleted=w404:dbl[])  [unwired: 1 out]
        n124 = Bundle By Name(cluster=w413, "Gate Start"=w421, "Gate Stop"=w420, "Gate Step (linear only)"=w419, "Gate Compliance"=w431, "Range mode"=w397, "Range"=w396) -> (w451:T3)
        n125 = Index Array(array=w404, index #1=0 ("Index")) -> (element #1=w416:dbl, element #2=w415:dbl, element #3=w414:dbl)  [unwired: 2 in]
        n126 = call <vilib>:"compatOverwrite.vi"("overwrite (F)"=TRUE) -> ("overwrite?"=w388:T7)
        n127 = Bundle By Name(cluster=w412, "Drain Start"=w416, "Drain Stop"=w415, "Drain Step"=w414, "Drain Compliance"=w432, "Range mode"=w395, "Range"=w398) -> (w450:T4)
        n128 = call "4155C Output.vi"("VISA resource name in"=w401, "Gate"=w451, "Drain"=w450, "Timings"=w430, "error in (no error)"=w400, "SMU4"=w390, "sweep mode"=w422, "Panel controls"=w452) -> ("VD"=w438:dbl[], "Outparams"=w393:T8, "VISA Resource Name out"=w428:refnum<visa-resource-name>, "IS"=w441:dbl[], "ID"=w440:dbl[], "IG"=w439:dbl[], "error out"=w429:errorcluster, "SMU4"=w389:dbl[])  [unwired: 12 in]
        n129 = Unbundle By Name(w393) -> ("V2 Step"=w394:dbl, "V2 Start"=w392:dbl, "Number of points"=w391:i32)
        n130 = Open/Create/Replace File(file path (use dialog)=w433, error in=w429, operation (0:open)=w388) -> (refnum out=w447:refnum<file>, error out=w448:errorcluster)  [unwired: 3 in, 1 out]
        n131 = call "4155C Make Big 2d array.vi"("1D Var1"=w438, "1d IS"=w441, "1d ID"=w440, "1d IG"=w439, "1d SMU4"=w389, "SMU4"=w390, "VAR2 START"=w392, "Number of VAR2 steps"=w391, "VAR2 STEP"=w394, "VAR1 Name"="Vd", "Decimal places in header"=i8 1, "VAR2 Name"="Vg") -> ("Header array"=w443:string[], "Data array"=w444:dbl[][])  [unwired: 14 in]
        n132 = call "4155C Write array to file.vi"("Byte Stream File Refnum"=w447, "Header"=w443, "Data Array"=w444, "error in (no error)"=w448) -> ("dup refnum"=w445:refnum<file>, "error out"=w446:errorcluster)  [unwired: 1 in]
        n133 = Close File(refnum=w445, error in=w446) -> (error out=w427:errorcluster)  [unwired: 1 out]
      }
      frame "output-fpp" {
        n134 = Number To Decimal String(number=w456) -> (decimal integer string=w510:string)  [unwired: 1 in]
        n135 = Bundle By Name(cluster=w486, "Emergency Stop"=w513) -> (w523:T6)
        n136 = Delete From Array(array=w501, index=0 ("Index")) -> (deleted portion=w499:string, array with subset deleted=w498:string[])  [unwired: 1 in]
        n137 = VISA Write(VISA resource name=w477, write buffer=":PAGE:CHAN:MODE SWE;" ("write buffer (\"\")"), error in (no error)=w474) -> (VISA resource name out=w476:refnum<visa-resource-name>, error out=w475:errorcluster)  [unwired: 1 out]
        n138 = Concatenate Strings(w509, "-outputfpp-" ("Substring"), w510, w455, ".txt" ("Substring")) -> (w512:string)
        n139 = case shown="\"d\", Default" w499 {
          tunnel: [w524 w525] -> w497
          frame "s" {
            w524 = u16 0 items=["Single", "Double"] ("sweep mode")
          }
          frame "d", Default {
            w525 = u16 1 items=["Single", "Double"] ("sweep mode")
          }
        }
        n140 = Fract/Exp String To Number(string=w498) -> (number=w480:dbl[])  [unwired: 3 in, 1 out]
        n141 = String To Path(string=w512) -> (path=w508:path)
        n142 = Index Array(array=w480, index #1=0 ("Index")) -> (element #1=w496:dbl, element #2=w495:dbl, element #3=w494:dbl)  [unwired: 2 in]
        n143 = Delete From Array(array=w480, length=3 ("Length"), index=0 ("Index")) -> (array with subset deleted=w479:dbl[])  [unwired: 1 out]
        n144 = Bundle By Name(cluster=w488, "Gate Start"=w496, "Gate Stop"=w495, "Gate Step (linear only)"=w494, "Gate Compliance"=w506, "Range mode"=w472, "Range"=w471) -> (w522:T3)
        n145 = Index Array(array=w479, index #1=0 ("Index")) -> (element #1=w491:dbl, element #2=w490:dbl, element #3=w489:dbl)  [unwired: 2 in]
        n146 = call <vilib>:"compatOverwrite.vi"("overwrite (F)"=TRUE) -> ("overwrite?"=w460:T7)
        n147 = Bundle By Name(cluster=w487, "Drain Start"=w491, "Drain Stop"=w490, "Drain Step"=w489, "Drain Compliance"=w507, "Range mode"=w470, "Range"=w473) -> (w521:T4)
        n148 = call "4155C Output-FPP.vi"("VISA resource name in"=w476, "Gate"=w522, "Drain"=w521, "Timings"=w505, "error in (no error)"=w475, "sweep mode"=w497, "Panel controls"=w523) -> ("VD"=w465:dbl[], "Outparams"=w468:T8, "VISA Resource Name out"=w503:refnum<visa-resource-name>, "Vprobe2"=w464:dbl[], "ID"=w463:dbl[], "IG"=w462:dbl[], "Vprobe1"=w461:dbl[], "error out"=w504:errorcluster)  [unwired: 13 in]
        n149 = Unbundle By Name(w468) -> ("V2 Step"=w469:dbl, "V2 Start"=w467:dbl, "Number of points"=w466:i32)
        n150 = Open/Create/Replace File(file path (use dialog)=w508, error in=w504, operation (0:open)=w460) -> (refnum out=w518:refnum<file>, error out=w519:errorcluster)  [unwired: 3 in, 1 out]
        n151 = call "4155C Make Big 2d array FPP.vi"("1D Var1"=w465, "1d ID"=w463, "1d Vp2"=w464, "1d IG"=w462, "1d Vp1"=w461, "VAR2 START"=w467, "Number of VAR2 steps"=w466, "VAR2 STEP"=w469, "VAR1 Name"="Vd", "Decimal places in header"=i8 1, "VAR2 Name"="Vg") -> ("Header array"=w514:string[], "Data array"=w515:dbl[][])  [unwired: 15 in]
        n152 = call "4155C Write array to file.vi"("Byte Stream File Refnum"=w518, "Header"=w514, "Data Array"=w515, "error in (no error)"=w519) -> ("dup refnum"=w516:refnum<file>, "error out"=w517:errorcluster)  [unwired: 1 in]
        n153 = Close File(refnum=w516, error in=w517) -> (error out=w502:errorcluster)  [unwired: 1 out]
      }
      frame "itime" {
        n154 = Delete From Array(array=w539, index=0 ("Index")) -> (deleted portion=w540:string)  [unwired: 1 in, 1 out]
        n155 = case shown="\"l\"" w540 {
          tunnel: w538 -> [w544 w546 w549]
          tunnel: [w543 w545 w548] -> w531
          frame "s" {
            w542 = u32 0 items=["short  ", "medium  ", "long  "] ("integration time 2")
            n156 = Bundle By Name(cluster=w544, "integration time"=w542) -> (w543:T5)
          }
          frame "m", Default {
            w547 = u32 1 items=["short  ", "medium  ", "long  "] ("integration time 2")
            n157 = Bundle By Name(cluster=w546, "integration time"=w547) -> (w545:T5)
          }
          frame "l" {
            w550 = u32 2 items=["short  ", "medium  ", "long  "] ("integration time 2")
            n158 = Bundle By Name(cluster=w549, "integration time"=w550) -> (w548:T5)
          }
        }
      }
      frame "pulsed" {
        n159 = Delete From Array(array=w565, index=0 ("Index")) -> (deleted portion=w566:string, array with subset deleted=w553:string[])  [unwired: 1 in]
        n160 = case shown="\"on\", Default" w566 {
          tunnel: w564 -> [w576 w579]
          tunnel: [w575 w578] -> w557
          tunnel: w553 -> [w573 _]
          frame "on", Default {
            w574 = u16 1 items=["Continuous", "Pulsed"] ("sweep method")
            n161 = Fract/Exp String To Number(string=w573) -> (number=w571:dbl[])  [unwired: 3 in, 1 out]
            n162 = Index Array(array=w571, index #1=0 ("Index")) -> (element #1=w570:dbl, element #2=w569:dbl, element #3=w568:dbl)  [unwired: 2 in]
            n163 = Bundle By Name(cluster=w576, "sweep method"=w574, "Pulse period"=w570, "Base voltage"=w569, "Pulse width"=w568) -> (w575:T5)
          }
          frame "off" {
            w577 = u16 0 items=["Continuous", "Pulsed"] ("sweep method")
            n164 = Bundle By Name(cluster=w579, "sweep method"=w577) -> (w578:T5)
          }
        }
      }
      frame "gaterangemode" {
        n165 = Delete From Array(array=w592, index=0 ("Index")) -> (deleted portion=w593:string)  [unwired: 1 in, 1 out]
        n166 = case shown="\"f\"" w593 {
          tunnel: [w595 w596 w597] -> w582
          frame "a", Default {
            w595 = u16 0 items=["Auto", "Limited", "Fixed"] ("Gate Range\nmode 2")
          }
          frame "f" {
            w596 = u16 2 items=["Auto", "Limited", "Fixed"] ("Gate Range\nmode 2")
          }
          frame "l" {
            w597 = u16 1 items=["Auto", "Limited", "Fixed"] ("Gate Range\nmode 2")
          }
        }
      }
      frame "gaterange" {
        (unwired) u8 11 items=["10fA  ", "100fA  ", "1nA  ", "10nA", "100nA", "1uA", "10uA", "100uA", "1mA", "10mA", "100mA", "1A"] ("Gate Range 2")
        n167 = Delete From Array(array=w617, index=0 ("Index")) -> (deleted portion=w607:string)  [unwired: 1 in, 1 out]
        n168 = Scan Value(string=w607, format string="") -> (value=w605:dbl)  [unwired: 1 in, 1 out]
        n169 = Logarithm Base 10(1:w605) -> (0:w604:dbl)
        n170 = Round To Nearest(number=w604) -> (nearest integer value=w603:dbl)
        n171 = Add(x=w603, y=11.0) -> (x+y=w601:dbl)
        n172 = To Unsigned Byte Integer(number=w601) -> (unsigned 8bit integer=w600:u8)
      }
      frame "drainrange" {
        (unwired) u8 11 items=["10fA  ", "100fA  ", "1nA  ", "10nA", "100nA", "1uA", "10uA", "100uA", "1mA", "10mA", "100mA", "1A"] ("Gate Range 2")
        n173 = Delete From Array(array=w638, index=0 ("Index")) -> (deleted portion=w629:string)  [unwired: 1 in, 1 out]
        n174 = Scan Value(string=w629, format string="") -> (value=w627:dbl)  [unwired: 1 in, 1 out]
        n175 = Logarithm Base 10(1:w627) -> (0:w626:dbl)
        n176 = Round To Nearest(number=w626) -> (nearest integer value=w625:dbl)
        n177 = Add(x=w625, y=11.0) -> (x+y=w623:dbl)
        n178 = To Unsigned Byte Integer(number=w623) -> (unsigned 8bit integer=w622:u8)
      }
      frame "drainrangemode" {
        n179 = Delete From Array(array=w652, index=0 ("Index")) -> (deleted portion=w653:string)  [unwired: 1 in, 1 out]
        n180 = case shown="\"f\"" w653 {
          tunnel: [w655 w656 w657] -> w642
          frame "a", Default {
            w655 = u16 0 items=["Auto", "Limited", "Fixed"] ("Gate Range\nmode 2")
          }
          frame "f" {
            w656 = u16 2 items=["Auto", "Limited", "Fixed"] ("Gate Range\nmode 2")
          }
          frame "l" {
            w657 = u16 1 items=["Auto", "Limited", "Fixed"] ("Gate Range\nmode 2")
          }
        }
      }
      frame "Error", Default {
      }
      frame "logfile" {
        n181 = Number To Decimal String(number=w672) -> (decimal integer string=w707:string)  [unwired: 1 in]
        n182 = Concatenate Strings(w706, "logfile" ("Substring"), w707, w670, ".txt" ("Substring")) -> (w704:string)
        n183 = String To Path(string=w704) -> (path=w677:path)
        n184 = Unbundle(w703) -> ("integration time"=w702:u32, "Short/Long integration time"=w701:dbl, "hold time (sec)"=w700:dbl, "delay time (sec)"=w699:dbl, "Step Time (0 disables)"=w698:dbl, "sweep method"=w697:u16, "Pulse period"=w696:dbl, "Base voltage"=w695:dbl, "Pulse width"=w694:dbl)
        n185 = Build Array(w702, w701, w700, w699, w698, w697, w696, w695, w694, w688, w689, w690, w691, w692, w693) -> (w681:dbl[])
        n186 = Insert Into Array(array=dbl[][] [] ("Input Array"), new element=w681) -> (w680:dbl[][])  [unwired: 2 in]
        n187 = call <vilib>:"compatOverwrite.vi"("overwrite (F)"=TRUE) -> ("overwrite?"=w675:T7)
        n188 = Open/Create/Replace File(file path (use dialog)=w677, error in=w679, operation (0:open)=w675) -> (refnum out=w685:refnum<file>, error out=w684:errorcluster)  [unwired: 3 in, 1 out]
        n189 = call "4155C Write array to file.vi"("Byte Stream File Refnum"=w685, "Header"=string[] ["Int Time", "Short/Long Itime", "Hold time", "Delay time", "Step time", "Sweep method", "Pulse period", "Base Voltage", "Pulse width", "Drain compliance", "Gate compliance", "Gate range mode", "Gate range", "S/D range mode", "S/D range"], "Data Array"=w680, "error in (no error)"=w684) -> ("dup refnum"=w687:refnum<file>, "error out"=w686:errorcluster)  [unwired: 1 in]
        n190 = Close File(refnum=w687, error in=w686) -> (error out=w678:errorcluster)  [unwired: 1 out]
      }
      frame "sample" {
        n191 = Number To Decimal String(number=w711) -> (decimal integer string=w759:string)  [unwired: 1 in]
        n192 = Fract/Exp String To Number(string=w756) -> (number=w717:dbl[])  [unwired: 3 in, 1 out]
        n193 = Concatenate Strings(w734, "-sample-" ("Substring"), w759, w709, ".txt" ("Substring")) -> (w757:string)
        n194 = String To Path(string=w757) -> (path=w738:path)
        n195 = Index Array(array=w717, index=0 ("Index")) -> (element=w754:dbl)
        n196 = Index Array(array=w717, index=2 ("Index")) -> (element=w750:dbl)
        n197 = Index Array(array=w717, index=3 ("Index")) -> (element=w719:dbl)
        n198 = Index Array(array=w717, index=4 ("Index")) -> (element=w716:dbl)
        n199 = call "4155C Config Sampling Measurements.vi"("Sampling interval"=w716, "Sample time"=w719, "Display on/off"=TRUE, "Timings"=w725, "Num Points"=w750, "error in (no error)"=w761, "Drain Compliance"=w760, "Gate Compliance"=w735, "VISA session"=w762) -> ("error out"=w763:errorcluster, "dup VISA resource name"=w764:refnum<visa-resource-name>)  [unwired: 1 in]
        n200 = Index Array(array=w717, index=1 ("Index")) -> (element=w751:dbl)
        n201 = call "4155C Take Sample.vi"("Emergency Stop"=w731, "error in (no error)"=w763, "Vd"=w751, "Vg"=w754, "VISA resource name in"=w764) -> ("error out"=w729:errorcluster, "Id"=w766:dbl[], "Ig"=w740:dbl[], "VISA Resource Name out"=w727:refnum<visa-resource-name>, "Is"=w765:dbl[], "Time"=w744:dbl[])  [unwired: 1 in]
        n202 = Insert Into Array(array=dbl[][] [] ("Input Array"), new element=w744) -> (w743:dbl[][])  [unwired: 2 in]
        n203 = Insert Into Array(array=w743, new element=w740) -> (w742:dbl[][])  [unwired: 2 in]
        n204 = Insert Into Array(array=w742, new element=w766) -> (w741:dbl[][])  [unwired: 2 in]
        n205 = VISA Write(VISA resource name=w727, write buffer=":DISP ON" ("write buffer (\"\")"), error in (no error)=w729) -> (VISA resource name out=w726:refnum<visa-resource-name>, error out=w728:errorcluster)  [unwired: 1 out]
        n206 = Insert Into Array(array=w741, new element=w765) -> (w733:dbl[][])  [unwired: 2 in]
        n207 = Transpose 2D Array(2D array=w733) -> (transposed array=w732:dbl[][])
        n208 = call <vilib>:"compatOverwrite.vi"("overwrite (F)"=TRUE) -> ("overwrite?"=w714:T7)
        n209 = Open/Create/Replace File(file path (use dialog)=w738, error in=w728, operation (0:open)=w714) -> (refnum out=w747:refnum<file>, error out=w746:errorcluster)  [unwired: 3 in, 1 out]
        n210 = call "4155C Write array to file.vi"("Byte Stream File Refnum"=w747, "Header"=string[] ["Time /s", "Ig /A", "Id /A", "Is /A"], "Data Array"=w732, "error in (no error)"=w746) -> ("dup refnum"=w749:refnum<file>, "error out"=w748:errorcluster)  [unwired: 1 in]
        n211 = Close File(refnum=w749, error in=w748) -> (error out=w736:errorcluster)  [unwired: 1 out]
      }
      frame "samplei" {
        n212 = Number To Decimal String(number=w768) -> (decimal integer string=w820:string)  [unwired: 1 in]
        n213 = Fract/Exp String To Number(string=w817) -> (number=w784:dbl[])  [unwired: 3 in, 1 out]
        n214 = Concatenate Strings(w799, "-samplei-" ("Substring"), w820, w767, ".txt" ("Substring")) -> (w818:string)
        n215 = String To Path(string=w818) -> (path=w802:path)
        n216 = Index Array(array=w784, index=4 ("Index")) -> (element=w778:dbl)
        n217 = Index Array(array=w784, index=3 ("Index")) -> (element=w779:dbl)
        n218 = Index Array(array=w784, index=1 ("Index")) -> (element=w781:dbl)
        n219 = Index Array(array=w784, index=0 ("Index")) -> (element=w782:dbl)
        n220 = Index Array(array=w784, index=2 ("Index")) -> (element=w780:dbl)
        n221 = call "4155C Config SamplingI Measurements.vi"("Sample time"=w780, "Display on/off"=TRUE, "Timings"=w791, "Num Points"=w781, "error in (no error)"=w822, "Sampling interval"=w779, "VISA session"=w823) -> ("error out"=w824:errorcluster, "dup VISA resource name"=w825:refnum<visa-resource-name>)  [unwired: 3 in]
        n222 = call "4155C Take SampleI.vi"("Emergency Stop"=w796, "error in (no error)"=w824, "Idg 2"=w782, "Vdg compliance 2"=w778, "VISA resource name in"=w825) -> ("error out"=w794:errorcluster, "Idg"=w827:dbl[], "Vdg"=w804:dbl[], "VISA Resource Name out"=w792:refnum<visa-resource-name>, "Is"=w826:dbl[], "Time"=w808:dbl[])  [unwired: 1 in]
        n223 = Insert Into Array(array=dbl[][] [] ("Input Array"), new element=w808) -> (w807:dbl[][])  [unwired: 2 in]
        n224 = Insert Into Array(array=w807, new element=w804) -> (w806:dbl[][])  [unwired: 2 in]
        n225 = Insert Into Array(array=w806, new element=w827) -> (w805:dbl[][])  [unwired: 2 in]
        n226 = VISA Write(VISA resource name=w792, write buffer=":DISP ON" ("write buffer (\"\")"), error in (no error)=w794) -> (VISA resource name out=w777:refnum<visa-resource-name>, error out=w793:errorcluster)  [unwired: 1 out]
        n227 = Insert Into Array(array=w805, new element=w826) -> (w798:dbl[][])  [unwired: 2 in]
        n228 = Transpose 2D Array(2D array=w798) -> (transposed array=w797:dbl[][])
        n229 = call <vilib>:"compatOverwrite.vi"("overwrite (F)"=TRUE) -> ("overwrite?"=w772:T7)
        n230 = Open/Create/Replace File(file path (use dialog)=w802, error in=w793, operation (0:open)=w772) -> (refnum out=w811:refnum<file>, error out=w810:errorcluster)  [unwired: 3 in, 1 out]
        n231 = call "4155C Write array to file.vi"("Byte Stream File Refnum"=w811, "Header"=string[] ["Time /s", "Vdg /V", "Idg /A", "Is /A"], "Data Array"=w797, "error in (no error)"=w810) -> ("dup refnum"=w813:refnum<file>, "error out"=w812:errorcluster)  [unwired: 1 in]
        n232 = Close File(refnum=w813, error in=w812) -> (error out=w775:errorcluster)  [unwired: 1 out]
        n233 = VISA Write(VISA resource name=w777, write buffer=";:PAGE:SCON:STAN OFF;:PAGE:CHAN:VSU2:DIS;" ("write buffer (\"\")"), error in (no error)=w775) -> (VISA resource name out=w773:refnum<visa-resource-name>, error out=w774:errorcluster)  [unwired: 1 out]
      }
      frame "#" {
        n234 = VISA Write(VISA resource name=w834, write buffer=":DISP ON" ("write buffer (\"\")"), error in (no error)=w833) -> (VISA resource name out=w832:refnum<visa-resource-name>, error out=w831:errorcluster)  [unwired: 1 out]
      }
      frame "stressV" {
        n235 = Number To Decimal String(number=w844) -> (decimal integer string=w885:string)  [unwired: 1 in]
        n236 = Fract/Exp String To Number(string=w882) -> (number=w855:dbl[])  [unwired: 3 in, 1 out]
        n237 = Concatenate Strings(w869, "-stressV-" ("Substring"), w885, w843, ".txt" ("Substring")) -> (w883:string)
        n238 = String To Path(string=w883) -> (path=w873:path)
        n239 = Index Array(array=w855, index=3 ("Index")) -> (element=w852:dbl)
        n240 = Index Array(array=w855, index=1 ("Index")) -> (element=w850:dbl)
        n241 = Index Array(array=w855, index=0 ("Index")) -> (element=w849:dbl)
        n242 = Index Array(array=w855, index=4 ("Index")) -> (element=w854:dbl)
        n243 = Index Array(array=w855, index=2 ("Index")) -> (element=w851:dbl)
        n244 = call "4155C Config V Stress.vi"("VISA session"=w888, "ID compliance"=w852, "VD"=w850, "VG"=w849, "IG compliance"=w851, "error in (no error)"=w887, "Display on/off"=TRUE) -> ("dup VISA resource name"=w890:refnum<visa-resource-name>, "error out"=w889:errorcluster)
        n245 = call "4155C Apply Stress.vi"("error in (no error)"=w889, "Duration"=w854, "Emergency Stop"=w868, "VISA resource name in"=w890) -> ("error out"=w866:errorcluster, "VISA Resource Name out"=w864:refnum<visa-resource-name>)
        n246 = VISA Write(VISA resource name=w864, write buffer=":DISP ON" ("write buffer (\"\")"), error in (no error)=w866) -> (VISA resource name out=w863:refnum<visa-resource-name>, error out=w865:errorcluster)  [unwired: 1 out]
        n247 = call <vilib>:"compatOverwrite.vi"("overwrite (F)"=TRUE) -> ("overwrite?"=w848:T7)
        n248 = Open/Create/Replace File(file path (use dialog)=w873, error in=w865, operation (0:open)=w848) -> (refnum out=w876:refnum<file>, error out=w875:errorcluster)  [unwired: 3 in, 1 out]
        n249 = call "4155C Write array to file.vi"("Byte Stream File Refnum"=w876, "Header"=string[] ["V stress completed successfully", ""], "error in (no error)"=w875) -> ("dup refnum"=w878:refnum<file>, "error out"=w877:errorcluster)  [unwired: 2 in]
        n250 = Close File(refnum=w878, error in=w877) -> (error out=w871:errorcluster)  [unwired: 1 out]
      }
      frame "stressI" {
        n251 = Number To Decimal String(number=w892) -> (decimal integer string=w929:string)  [unwired: 1 in]
        n252 = Fract/Exp String To Number(string=w926) -> (number=w901:dbl[])  [unwired: 3 in, 1 out]
        n253 = Concatenate Strings(w913, "-stressI-" ("Substring"), w929, w891, ".txt" ("Substring")) -> (w927:string)
        n254 = String To Path(string=w927) -> (path=w917:path)
        n255 = Index Array(array=w901, index=1 ("Index")) -> (element=w897:dbl)
        n256 = Index Array(array=w901, index=0 ("Index")) -> (element=w898:dbl)
        n257 = call "4155C Config I Stress.vi"("VISA session"=w932, "IDG"=w898, "VDG compliance"=w897, "error in (no error)"=w931, "Display on/off"=TRUE) -> ("dup VISA resource name"=w934:refnum<visa-resource-name>, "error out"=w933:errorcluster)
        n258 = Index Array(array=w901, index=2 ("Index")) -> (element=w899:dbl)
        n259 = call "4155C Apply Stress.vi"("error in (no error)"=w933, "Duration"=w899, "Emergency Stop"=w912, "VISA resource name in"=w934) -> ("error out"=w910:errorcluster, "VISA Resource Name out"=w908:refnum<visa-resource-name>)
        n260 = VISA Write(VISA resource name=w908, write buffer=":DISP ON" ("write buffer (\"\")"), error in (no error)=w910) -> (VISA resource name out=w907:refnum<visa-resource-name>, error out=w909:errorcluster)  [unwired: 1 out]
        n261 = call <vilib>:"compatOverwrite.vi"("overwrite (F)"=TRUE) -> ("overwrite?"=w896:T7)
        n262 = Open/Create/Replace File(file path (use dialog)=w917, error in=w909, operation (0:open)=w896) -> (refnum out=w920:refnum<file>, error out=w919:errorcluster)  [unwired: 3 in, 1 out]
        n263 = call "4155C Write array to file.vi"("Byte Stream File Refnum"=w920, "Header"=string[] ["I stress completed successfully", ""], "error in (no error)"=w919) -> ("dup refnum"=w922:refnum<file>, "error out"=w921:errorcluster)  [unwired: 2 in]
        n264 = Close File(refnum=w922, error in=w921) -> (error out=w915:errorcluster)  [unwired: 1 out]
      }
      frame "vsu2pulse" {
        n265 = Number To Decimal String(number=w936) -> (decimal integer string=w971:string)  [unwired: 1 in]
        n266 = Fract/Exp String To Number(string=w968) -> (number=w944:dbl[])  [unwired: 3 in, 1 out]
        n267 = Concatenate Strings(w956, "-vsu2-" ("Substring"), w971, w935, ".txt" ("Substring")) -> (w969:string)
        n268 = String To Path(string=w969) -> (path=w960:path)
        n269 = Index Array(array=w944, index=1 ("Index")) -> (element=w943:dbl)
        n270 = Index Array(array=w944, index=0 ("Index")) -> (element=w941:dbl)
        n271 = call "4155C Config VSU2 Stress.vi"("error in (no error)"=w973, "VSU2"=w941, "Display on/off"=TRUE, "VISA session"=w974) -> ("error out"=w975:errorcluster, "dup VISA resource name"=w976:refnum<visa-resource-name>)
        n272 = call "4155C Apply Stress.vi"("error in (no error)"=w975, "Duration"=w943, "Emergency Stop"=w955, "VISA resource name in"=w976) -> ("error out"=w953:errorcluster, "VISA Resource Name out"=w951:refnum<visa-resource-name>)
        n273 = VISA Write(VISA resource name=w951, write buffer=":DISP ON" ("write buffer (\"\")"), error in (no error)=w953) -> (VISA resource name out=w950:refnum<visa-resource-name>, error out=w952:errorcluster)  [unwired: 1 out]
        n274 = call <vilib>:"compatOverwrite.vi"("overwrite (F)"=TRUE) -> ("overwrite?"=w940:T7)
        n275 = Open/Create/Replace File(file path (use dialog)=w960, error in=w952, operation (0:open)=w940) -> (refnum out=w963:refnum<file>, error out=w962:errorcluster)  [unwired: 3 in, 1 out]
        n276 = call "4155C Write array to file.vi"("Byte Stream File Refnum"=w963, "Header"=string[] ["VSU2 pulse completed successfully", ""], "error in (no error)"=w962) -> ("dup refnum"=w965:refnum<file>, "error out"=w964:errorcluster)  [unwired: 2 in]
        n277 = Close File(refnum=w965, error in=w964) -> (error out=w958:errorcluster)  [unwired: 1 out]
      }
      frame "sample-fpp" {
        w989 = string[] ["Time /s", "Id VgVd /A", "Ig VgVd /A", "Vp1 VgVd /V", "Vp2 VgVd /V"] ("Header")
        w993 = "%d" ("format string")
        n278 = Number To Decimal String(number=w978) -> (decimal integer string=w1041:string)  [unwired: 1 in]
        n279 = Fract/Exp String To Number(string=w1038) -> (number=w1026:dbl[])  [unwired: 3 in, 1 out]
        n280 = Concatenate Strings(w1032, "-samplefpp-" ("Substring"), w1041, w977, ".txt" ("Substring")) -> (w1039:string)
        n281 = String To Path(string=w1039) -> (path=w1001:path)
        n282 = Index Array(array=w1026, index=0 ("Index")) -> (element=w987:dbl)
        n283 = Index Array(array=w1026, index=1 ("Index")) -> (element=w986:dbl)
        n284 = Index Array(array=w1026, index=2 ("Index")) -> (element=w1034:dbl)
        n285 = Index Array(array=w1026, index=3 ("Index")) -> (element=w1024:dbl)
        n286 = call "4155C Config Sampling Measurements FPP.vi"("VISA session"=w1044, "Num Points"=w1034, "Vg"=w987, "Display on/off"=TRUE, "Gate Compliance"=w1033, "Drain Compliance"=w1042, "Standby"="Standby", "error in (no error)"=w1043, "Timings"=w1031, "Vd"=w986, "Sample time"=w1024) -> ("dup VISA resource name"=w1003:refnum<visa-resource-name>, "error out"=w1002:errorcluster)  [unwired: 3 in]
        n287 = Number To Decimal String(number=w987) -> (decimal integer string=w1013:string)  [unwired: 1 in]
        n288 = call "4155C Take Sample FPP.vi"("VISA resource name in"=w1003, "error in (no error)"=w1002, "Emergency Stop"=w1004) -> ("Time"=w1008:dbl[], "Vp1"=w1018:dbl[], "VISA Resource Name out"=w984:refnum<visa-resource-name>, "Ig"=w1006:dbl[], "Id"=w1007:dbl[], "Vp2"=w1016:dbl[], "error out"=w1005:errorcluster)  [unwired: 10 in]
        n289 = Insert Into Array(array=dbl[][] [] ("Input Array"), new element=w1008) -> (w1022:dbl[][])  [unwired: 2 in]
        n290 = Number To Decimal String(number=w986) -> (decimal integer string=w1011:string)  [unwired: 1 in]
        n291 = Insert Into Array(array=w1022, new element=w1007) -> (w1021:dbl[][])  [unwired: 2 in]
        n292 = Concatenate Strings("(Vg = " ("Substring"), w1013, "V, Vd = " ("Substring"), w1011, "V)" ("Substring")) -> (w1009:string)
        n293 = Insert Into Array(array=w1021, new element=w1006) -> (w1020:dbl[][])  [unwired: 2 in]
        n294 = Insert Into Array(array=w1020, new element=w1018) -> (w1017:dbl[][])  [unwired: 2 in]
        n295 = Insert Into Array(array=w1017, new element=w1016) -> (w985:dbl[][])  [unwired: 2 in]
        n296 = call <vilib>:"compatOverwrite.vi"("overwrite (F)"=TRUE) -> ("overwrite?"=w982:T7)
        n297 = Open/Create/Replace File(file path (use dialog)=w1001, error in=w1005, operation (0:open)=w982) -> (refnum out=w998:refnum<file>, error out=w999:errorcluster)  [unwired: 3 in, 1 out]
        n298 = Array To Spreadsheet String(array=w989, 3:w993) -> (spreadsheet string=w995:string)  [unwired: 1 in]
        n299 = Transpose 2D Array(2D array=w985) -> (transposed array=w1015:dbl[][])
        n300 = Search and Replace String(replace all?=TRUE ("replace all? (F)"), input string=w995, search string="VgVd", replace string=w1009) -> (result string=w991:string)  [unwired: 4 in, 3 out]
        n301 = Spreadsheet String To Array(format string=w993, spreadsheet string=w991, array type (2D Dbl)=w989) -> (array=w990:string[])  [unwired: 1 in]
        n302 = call "4155C Write array to file.vi"("Byte Stream File Refnum"=w998, "Header"=w990, "Data Array"=w1015, "error in (no error)"=w999) -> ("dup refnum"=w996:refnum<file>, "error out"=w997:errorcluster)  [unwired: 1 in]
        n303 = Close File(refnum=w996, error in=w997) -> (error out=w983:errorcluster)  [unwired: 1 out]
      }
      frame "resample-fpp" {
        w1059 = string[] ["Time /s", "Id VgVd /A", "Ig VgVd /A", "Vp1 VgVd /V", "Vp2 VgVd /V"] ("Header")
        w1063 = "%d" ("format string")
        n304 = Number To Decimal String(number=w1045) -> (decimal integer string=w1103:string)  [unwired: 1 in]
        n305 = Fract/Exp String To Number(string=w1100) -> (number=w1052:dbl[])  [unwired: 3 in, 1 out]
        n306 = Concatenate Strings(w1096, "-resamplefpp-" ("Substring"), w1103, w1046, ".txt" ("Substring")) -> (w1101:string)
        n307 = String To Path(string=w1101) -> (path=w1071:path)
        n308 = Index Array(array=w1052, index=0 ("Index")) -> (element=w1058:dbl)
        n309 = Index Array(array=w1052, index=1 ("Index")) -> (element=w1057:dbl)
        n310 = Number To Decimal String(number=w1058) -> (decimal integer string=w1081:string)  [unwired: 1 in]
        n311 = call "4155C Take Sample FPP.vi"("VISA resource name in"=w1054, "error in (no error)"=w1053, "Emergency Stop"=w1072) -> ("Time"=w1076:dbl[], "Vp1"=w1086:dbl[], "VISA Resource Name out"=w1056:refnum<visa-resource-name>, "Ig"=w1074:dbl[], "Id"=w1075:dbl[], "Vp2"=w1084:dbl[], "error out"=w1073:errorcluster)  [unwired: 10 in]
        n312 = Insert Into Array(array=dbl[][] [] ("Input Array"), new element=w1076) -> (w1090:dbl[][])  [unwired: 2 in]
        n313 = Number To Decimal String(number=w1057) -> (decimal integer string=w1079:string)  [unwired: 1 in]
        n314 = Insert Into Array(array=w1090, new element=w1075) -> (w1089:dbl[][])  [unwired: 2 in]
        n315 = Concatenate Strings("(Vg = " ("Substring"), w1081, "V, Vd = " ("Substring"), w1079, "V)" ("Substring")) -> (w1077:string)
        n316 = Insert Into Array(array=w1089, new element=w1074) -> (w1088:dbl[][])  [unwired: 2 in]
        n317 = Insert Into Array(array=w1088, new element=w1086) -> (w1085:dbl[][])  [unwired: 2 in]
        n318 = Insert Into Array(array=w1085, new element=w1084) -> (w1051:dbl[][])  [unwired: 2 in]
        n319 = call <vilib>:"compatOverwrite.vi"("overwrite (F)"=TRUE) -> ("overwrite?"=w1050:T7)
        n320 = Open/Create/Replace File(file path (use dialog)=w1071, error in=w1073, operation (0:open)=w1050) -> (refnum out=w1068:refnum<file>, error out=w1069:errorcluster)  [unwired: 3 in, 1 out]
        n321 = Array To Spreadsheet String(array=w1059, 3:w1063) -> (spreadsheet string=w1065:string)  [unwired: 1 in]
        n322 = Transpose 2D Array(2D array=w1051) -> (transposed array=w1083:dbl[][])
        n323 = Search and Replace String(replace all?=TRUE ("replace all? (F)"), input string=w1065, search string="VgVd", replace string=w1077) -> (result string=w1061:string)  [unwired: 4 in, 3 out]
        n324 = Spreadsheet String To Array(format string=w1063, spreadsheet string=w1061, array type (2D Dbl)=w1059) -> (array=w1060:string[])  [unwired: 1 in]
        n325 = call "4155C Write array to file.vi"("Byte Stream File Refnum"=w1068, "Header"=w1060, "Data Array"=w1083, "error in (no error)"=w1069) -> ("dup refnum"=w1066:refnum<file>, "error out"=w1067:errorcluster)  [unwired: 1 in]
        n326 = Close File(refnum=w1066, error in=w1067) -> (error out=w1055:errorcluster)  [unwired: 1 out]
      }
      frame "serial" {
        n327 = Index Array(array=w1107, index=0 ("Index")) -> (element=w1106:string)
        n328 = call "Serial write and read v0.4.vi"("Termination char\n(0xA = '\\n' = LF)\n(0xD = '\\r' = CR)"="Termination char\n(0xA = '\\n' = LF)\n(0xD = '\\r' = CR)", "Enable Termination\nChar (T)"="Enable Termination\nChar (T)", "parity"="parity", "stop bits"="stop bits", "string to write"=w1106, "flow control"="flow control", "byte count"="byte count", "Serial Settings:Serial End Mode for Reads"="Serial Settings:Serial End Mode for Reads", "Timeout (ms)"="Timeout (ms)", "error in (no error)"=w1112, "VISA resource name"="VISA resource name", "baud rate"="baud rate", "data bits"="data bits") -> ("read string"=→"Serial output":string, "error out"=w1111:errorcluster)  [unwired: 1 in]
      }
    }
    "Line running" <- w46
    "Total iterations" <- w45
  }
  "error out" <- w9
